vi "EC_Applied_Motion_SXSYSZ_20170419A_3chNoBK.vi"() -> ()   [LabVIEW 2015]
uses:
  <vilib>/Instr/_visa.llb/VISA Configure Serial Port (Instr).vi
  <userlib>/caLab/Private/Put_DBL-1D_PV-1D.vi
  <userlib>/caLab/Private/Put_DBL_PV.vi
  <userlib>/caLab/Private/Get_PV-1D.vi
  <vilib>/Utility/file.llb/Write To Spreadsheet File (I64).vi
  <vilib>/Utility/file.llb/Read From Spreadsheet File (I64).vi
panel:
  out "x*2^n":dbl
  out "Jog Z4-":bool
  out "Jog Z4+":bool
  in  "Jog Z-- CNTL":bool
  in  "Jog Z++ CNTL":bool
  in  "Local":bool
  out "Movex4Z REQ":bool
  in  "Reset Jog counts":bool
  in  "Jog Z- CNTL":bool
  in  "Jog Z+ CNTL":bool
  in  "Jog Y- CNTL":bool
  in  "Jog Y+ CNTL":bool
  in  "Jog X- CNTL":bool
  in  "Jog X+ CNTL":bool
  out "APX:FZ_DOWN":dbl
  out "APX:FZ_UP":dbl
  out "APX:FY_DOWN":dbl
  out "APX:FY_UP":dbl
  out "APX:FX_DOWN":dbl
  out "APX:FX_UP":dbl
  out "FZ Jog Counts In Range?":bool
  out "FY Jog Counts In Range?":bool
  out "FX Jog Counts In Range?":bool
  in  "FZ Jog counts":i8
  in  "FY Jog counts":i8
  in  "FX Jog counts":i8
  in  "Dev 5 Voltage SW":bool=TRUE
  out "Isolated from GND?":bool
  in  "Crash Override":bool
  out "Dev5 Voltage PV":dbl
  in  "APX:FZabs":dbl
  in  "Move x4Z":bool
  out "Jog Z-":bool
  out "Jog X-":bool
  out "Jog Y-":bool
  out "Z Velocity MV mm/sec":dbl format="%.3f"
  out "Z Position MV mm":dbl
  out "Y Velocity MV mm/sec":dbl format="%.3f"
  out "Y Position MV mm":dbl
  out "X Velocity MV mm/sec":dbl format="%.3f"
  out "X Position MV mm":dbl
  in  "stop":bool
  in  "Tab Control 3":enum32{"Status", "Reset"}(tab)
  out "Y in Range":bool
  out "Y in Motion":bool
  out "X  in Range":bool
  out "X  in Motion":bool
  out "Z in Range":bool
  out "Z in Motion":bool
  out "X Ready":bool
  out "Y Ready":bool
  out "Z Ready":bool
  in  "Reset Y Position mm":dbl
  out "Reset Y Motor Steps":i32
  in  "Reset X Position mm":dbl
  out "Reset X Motor Steps":i32
  in  "Reset Z Position mm":dbl
  out "Reset Z Motor Steps":i32
  in  "Reset":bool
  in  "Tab Control":enum32{"mm", "preset", "step"}(tab)
  in  "APX:FXstep":dbl=0.1 min=0.1 max=0.2
  in  "FX Velocity SP mm/sec":dbl=0.010583500000000001
  in  "APX:FYstep":dbl=0.025 min=0.025 max=0.1
  in  "FY Velocity SP mm/sec":dbl=0.010583500000000001
  in  "APX:Fzstep":dbl=0.1 min=0.05 max=0.2
  in  "FZ Velocity SP mm/sec":dbl=0.0635
  in  "Z Jog Set":bool
  in  "Y Jog Set":bool
  in  "X Jog Set":bool
  in  "X Velocity SP step/sec":i32 min=1 max=1000
  in  "Y Velocity SP step/sec":i32 min=1 max=1000
  in  "Z Velocity SP step/sec":i32 min=1 max=500
  in  "Y Step SP":i32=-20000 min=-800000 max=800000 step=500
  in  "X Step SP":i32=-20000 min=-750000 max=750000 step=500
  in  "Z Step SP":i32=-20000 min=-3000 max=102400000 step=500
  out "X Step PV":i32 max=2000
  out "Y Step PV":i32 max=2000
  out "Z Step PV":i32 max=2000
  out "R Step PV":i32 max=2000
  out "Z COM PORT":refnum<visa-resource-name>="COM5"
  out "Z Holding Current %":i32
  out "Z Run Current %":i32
  out "Z offset mm":dbl
  out "Z mm/rev":dbl
  out "Z steps/rev":u32
  out "Z  velocity PV step/sec":i32
  out "Z MINPOS":i32=-94296
  out "Z MAXPOS":i32=-34296
  out "Jog Z+":bool
  out "Z Position mm PV":dbl
  out "X Position mm PV":dbl
  out "X velocity PV step/sec":i32
  out "Jog X+":bool
  out "X Holding Current %":i32
  out "X Run Current %":i32
  out "X offset mm":dbl
  out "X mm/rev":dbl
  out "X steps/rev":u32
  out "X MAXPOS":i32=-34296
  out "X MINPOS":i32=-94296
  out "X COM PORT":refnum<visa-resource-name>="COM5"
  out "Y Holding Current %":i32
  out "Y Run Current %":i32
  out "Y Position mm PV":dbl
  out "Y offset mm":dbl
  out "Y mm/rev":dbl
  out "Y steps/rev":u32
  out "Y velocity PV step/sec":i32
  in  "Stop":bool
  out "Jog Y+":bool
  out "Y MINPOS":i32=-94296
  out "Y MAXPOS":i32=-34296
  out "Y COM PORT":refnum<visa-resource-name>="COM5"
  # "APX:FY"
  # "Sample posiitoning EPICS"
  # "x-ray"
  # "APX:FZ"
  # "APX:FX"
  # "SPEAR"
  # "APX:FinePos"
  # "Stage"
  # "Current position"
  # "Jog step/velovity"
  # "sample to SSRL"
  # "FX"
  # "FY"
  # "FZ"
  # "R,L = green"
  # "L"
  # "M"
  # "R"
  # "Preset position"
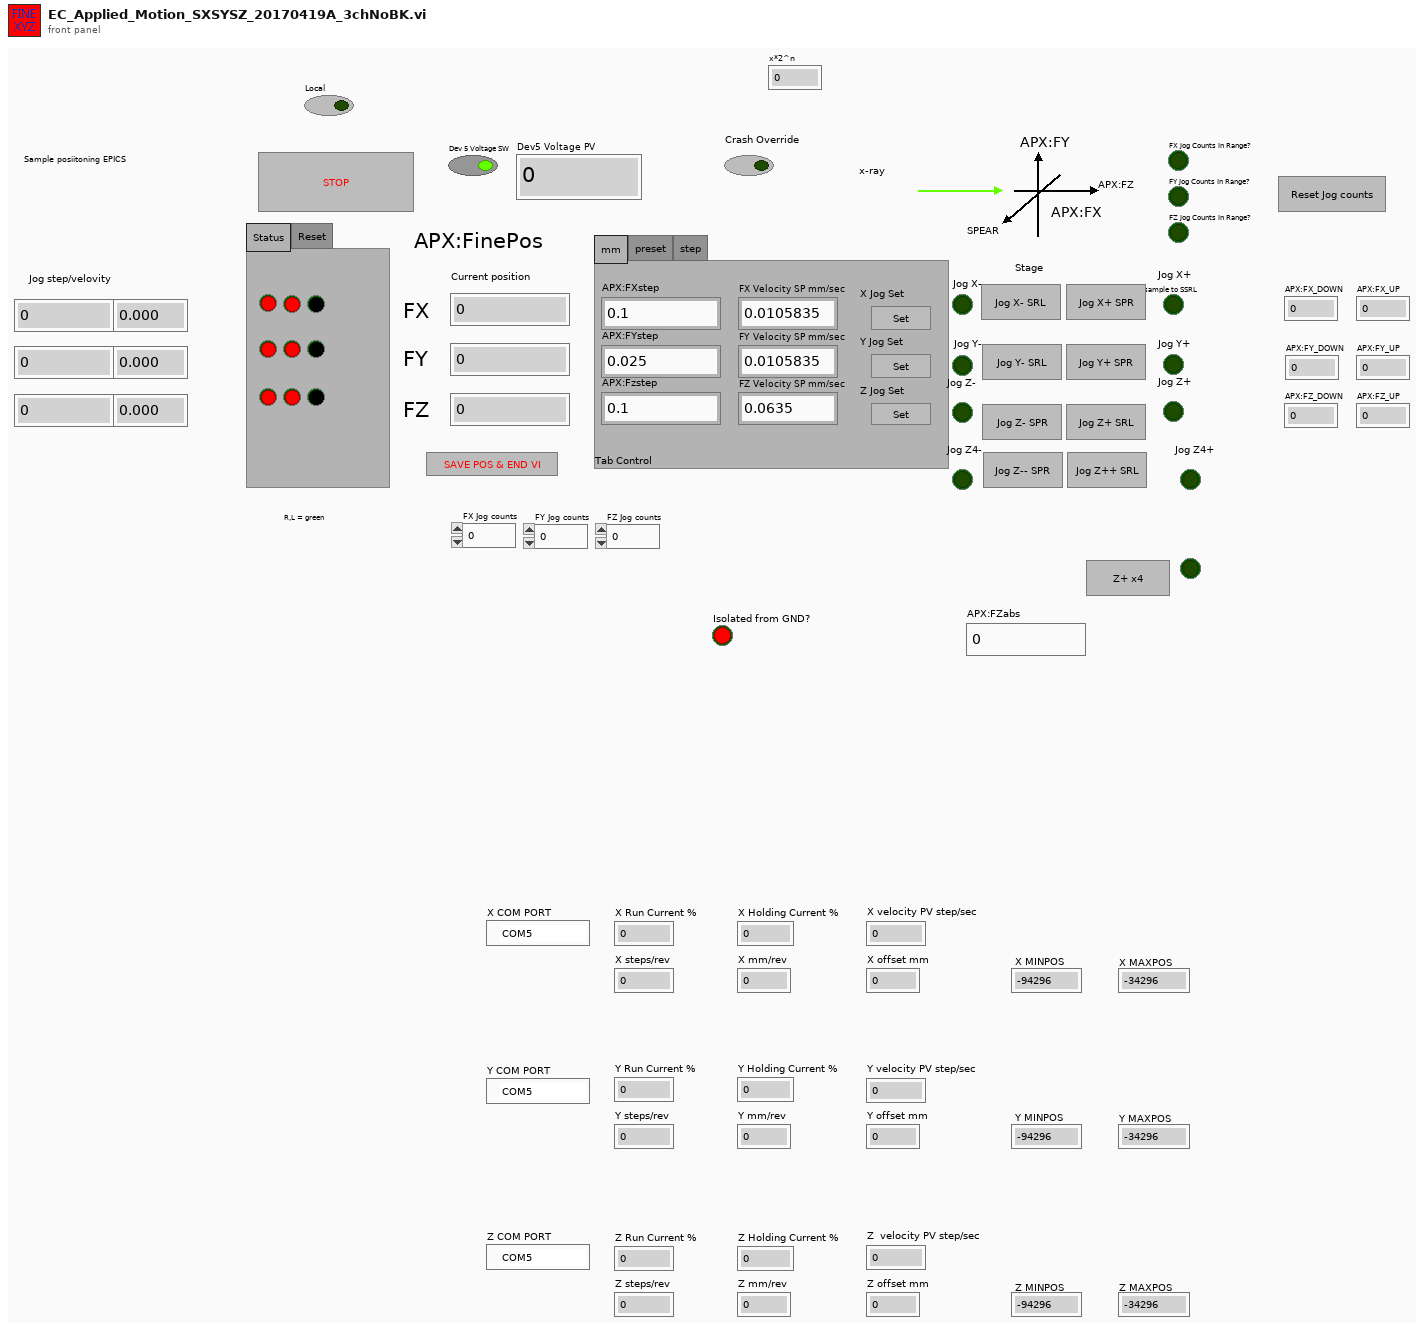
[diagram p1: front panel]
types:
  T1 = enum16{"Power-up Signature", "Accel Rate", "Accel Max", "Bit Rate", "Buffer Status", "Change Current", "Commence Jogging", "Change Jog Speed", "Continue", "Define Address", "Distance for FC,FM,FO,FY", "Decel Rate", "Distance or Position", "Define Limits", "Encoder Deadband", "Encoder Function", "Encoder Position", "Encoder Ratio", "Feed to Length with Speed Change", "Feed to Length", "Feed to Sensor with Mask Dist", "Feed to Length & Set Output", "Feed to Position", "Feed to Sensor", "Feed to Sensor w/safety", "Follow Handwheel", "Immediate Distance?", "Immediate Encoder?", "Immediate Low Output", "Immediate High Output", "Immediate Position?", "Input Status?", "Jog Accel/Decel", "Jog Disable", "Jog Enable", "Jog Speed", "Motor Disable", "Motor Enable", "Microstep Resolution", "Power up Current", "Power up Mode", "Pause", "Request Status", "Revision Level?", "Seek Home", "Stop Jogging", "Stop & Kill Buffer", "Set Output", "Set ABS Position", "Send String", "Stop", "Velocity for Speed Change", "Velocity Setting", "Wait for Input", "Wait Time"}
  T2 = enum8{"Enabled", "Disabled", "Disabled and Grayed Out"}
  T3 = cluster{"first row[0]":i64, "first row[1]":i64, "first row[2]":i64, "first row[3]":i64, "first row[4]":i64, "first row[5]":i64, "first row[6]":i64, "first row[7]":i64, "first row[8]":i64}
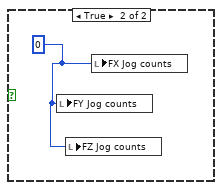
[diagram p5: hidden frame]
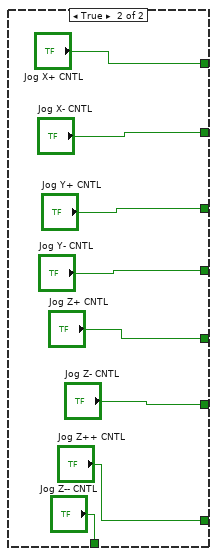
[diagram p7: hidden frame]
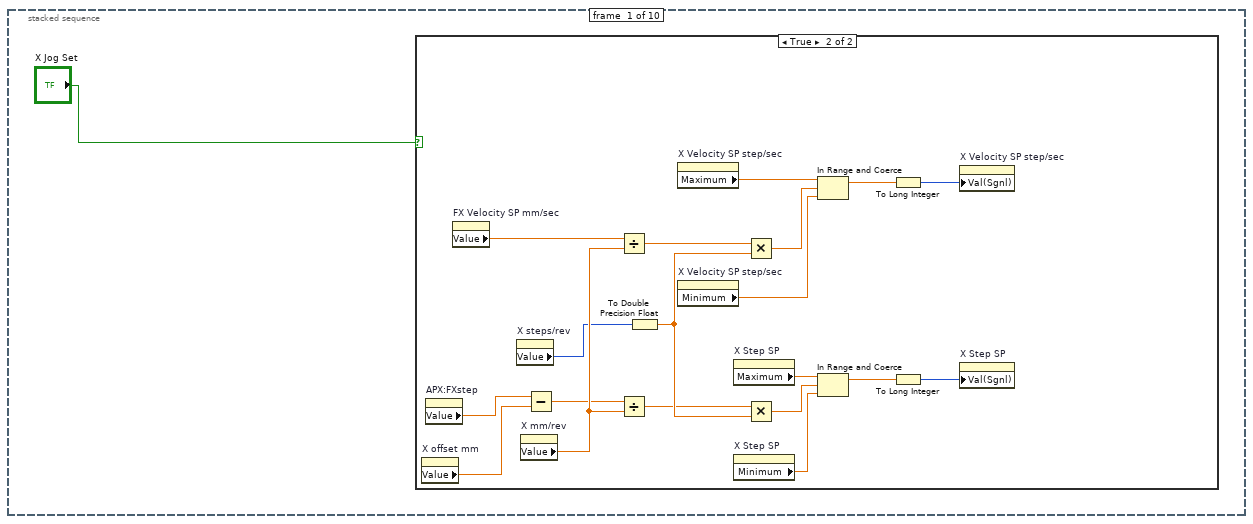
[diagram p8: hidden frame]
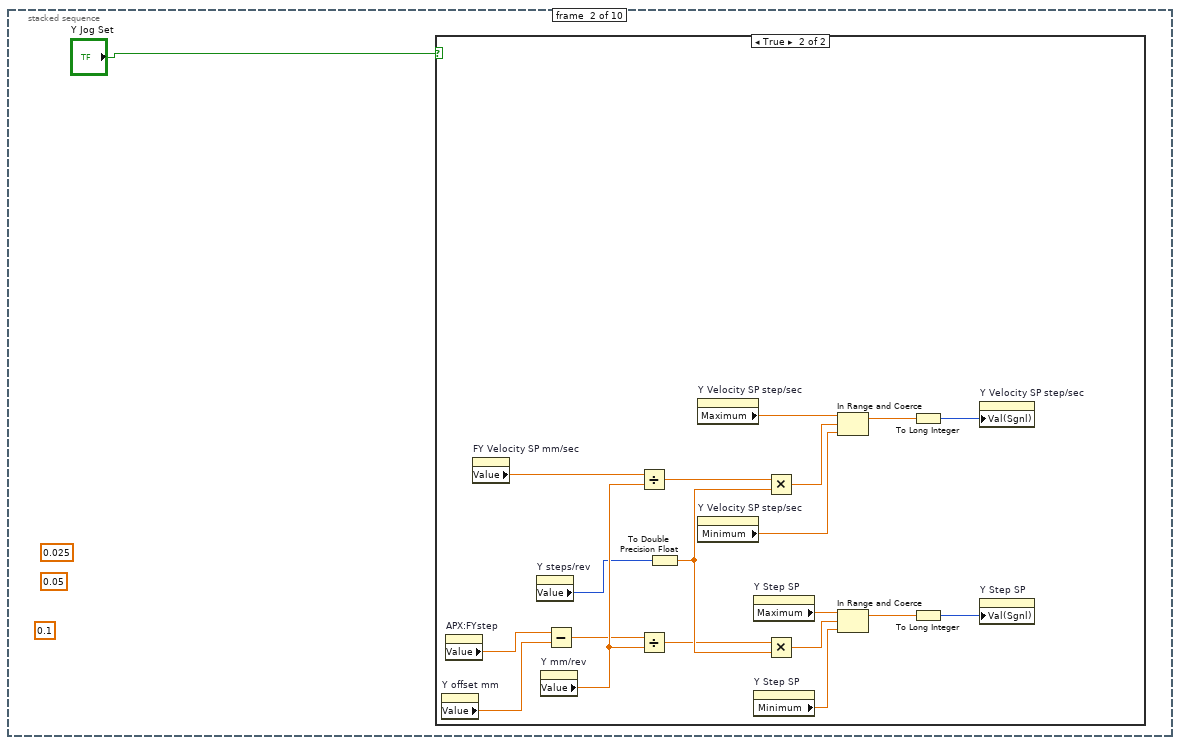
[diagram p10: hidden frame]
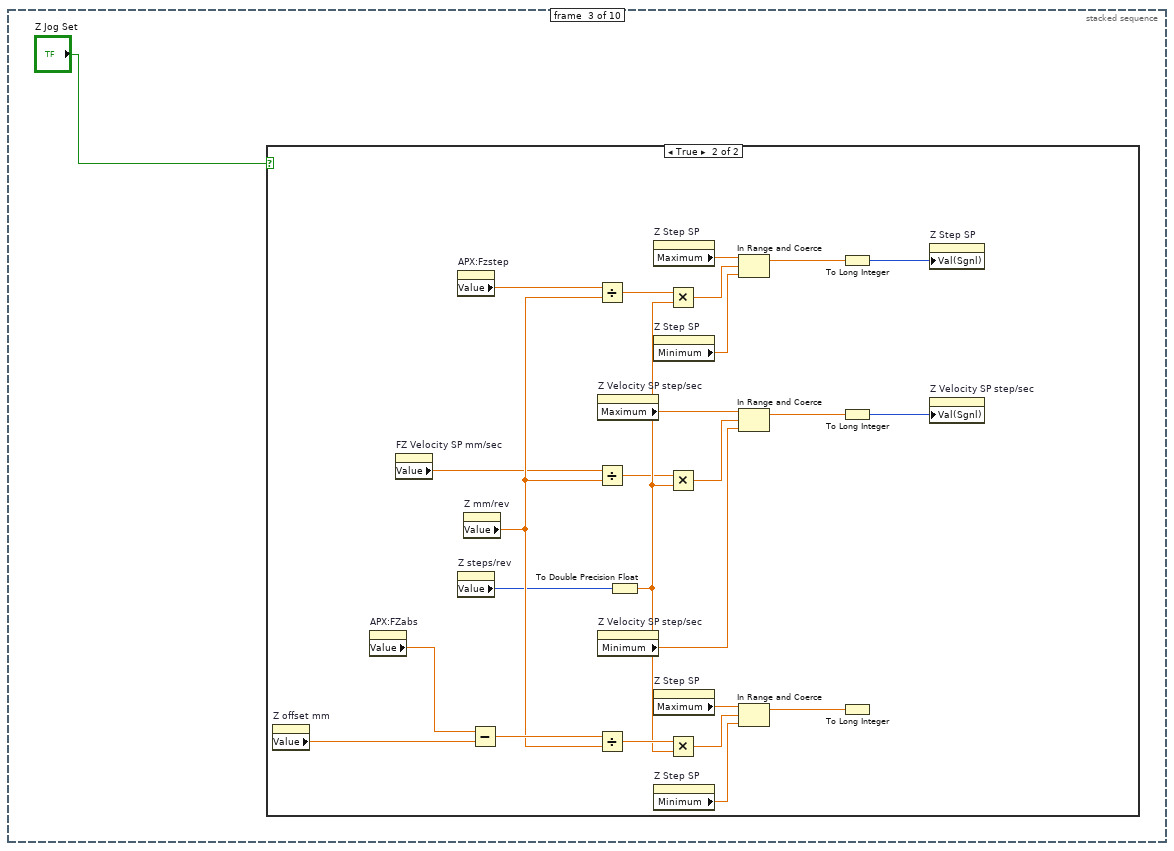
[diagram p12: hidden frame]
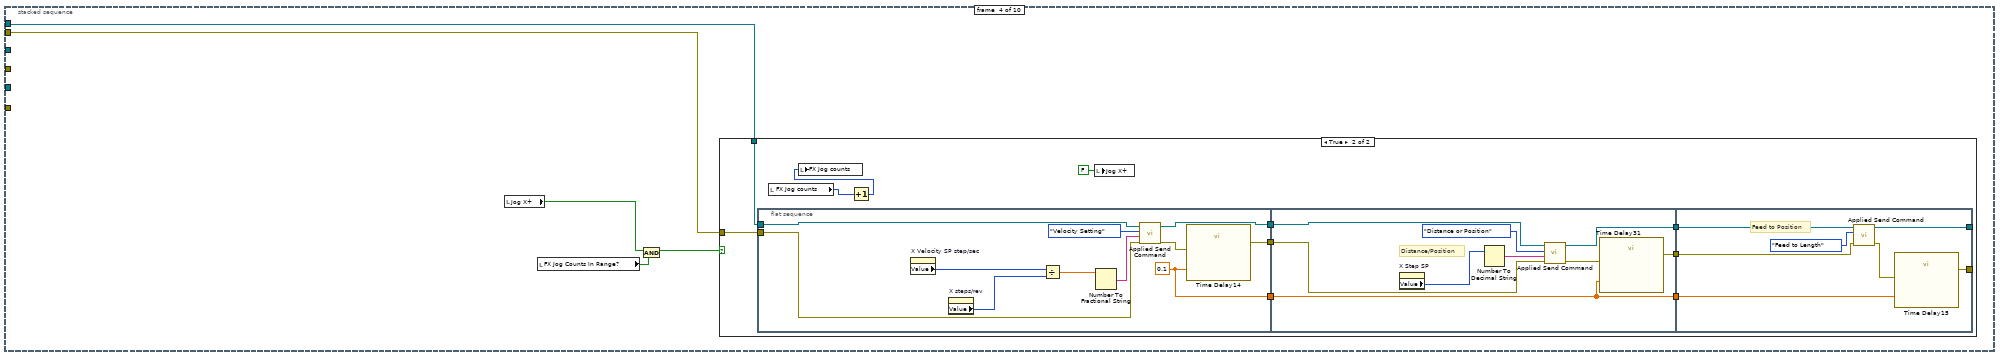
[diagram p14: hidden frame]
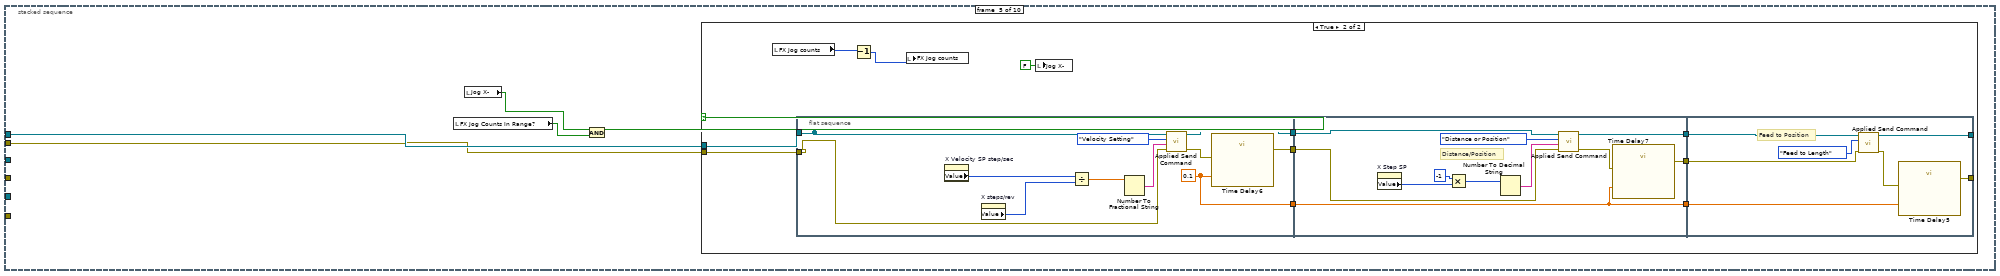
[diagram p16: hidden frame]
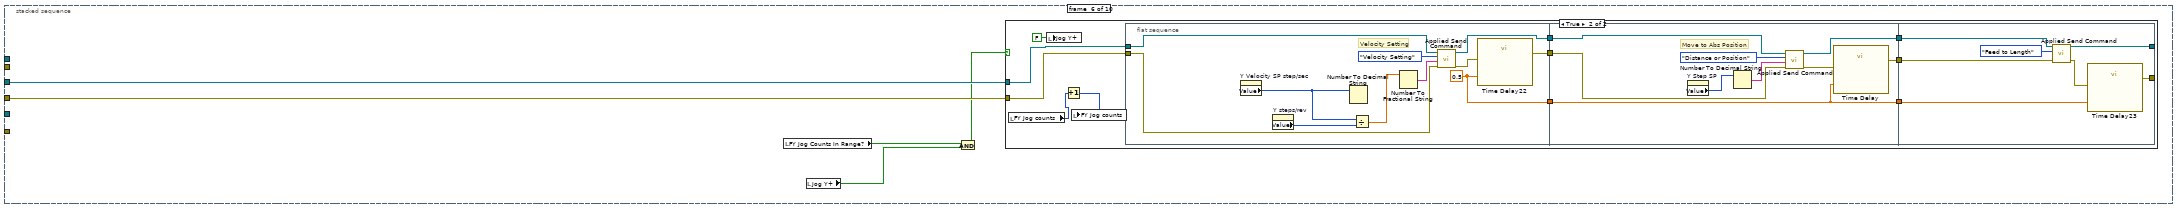
[diagram p18: hidden frame]
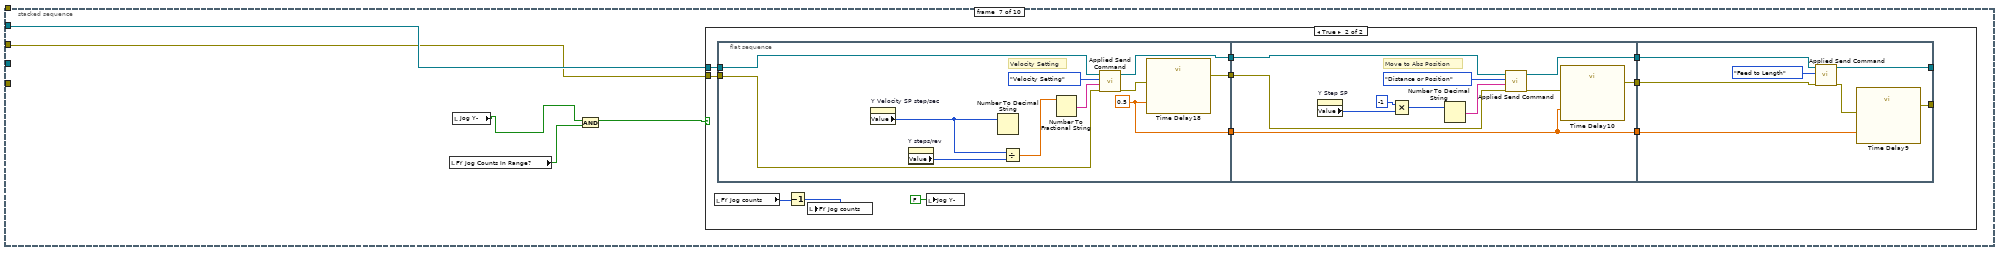
[diagram p20: hidden frame]
diagram:
  (unwired) FALSE
  n1 = flat-sequence {
    tunnel: [w58] -> w18
    tunnel: [w57] -> w17
    tunnel: w18 -> [w75]
    tunnel: w17 -> [w74]
    tunnel: [w73] -> w16
    tunnel: [w72] -> w15
    tunnel: [w78] -> w40
    tunnel: w16 -> [w86]
    tunnel: w15 -> [w85]
    tunnel: [w79] -> w14
    tunnel: w40 -> [w100]
    tunnel: [w99] -> w34
    tunnel: [w97] -> w33
    tunnel: [w102] -> w32
    tunnel: w14 -> [w101]
    tunnel: [w108] -> w38
    tunnel: [w109] -> w39
    tunnel: w34 -> [w109]
    tunnel: w33 -> [w108]
    tunnel: w32 -> [w107]
    frame #0 {
      "X Run Current %" <- 100 ("Run Current %")
      "X Holding Current %" <- 50 ("Holding Current %")
    }
    frame #1 {
      w45 = T2."Enabled" ("Disabled")
      n2 = property on="Jog X+" class="Bool"("DisabledEnum"=w45) -> ()  [unwired: 2 in, 2 out]
      n3 = property on="Jog X-" class="Bool"("DisabledEnum"=w45) -> ()  [unwired: 2 in, 2 out]
      n4 = property on="Jog Y+" class="Bool"("DisabledEnum"=w45) -> ()  [unwired: 2 in, 2 out]
      n5 = property on="Jog Z+" class="Bool"("DisabledEnum"=w45) -> ()  [unwired: 2 in, 2 out]
      n6 = property on="Jog Y-" class="Bool"("DisabledEnum"=w45) -> ()  [unwired: 2 in, 2 out]
      n7 = property on="Jog Z-" class="Bool"("DisabledEnum"=w45) -> ()  [unwired: 2 in, 2 out]
    }
    frame #2 {
      w48 = 0.21167 ("MM/rev")
      w51 = u32 20000 ("step/rev")
      w46 = 1000 ("Value (Signaling)")
      (unwired) 0.01 ("Value (Signaling)")
      n8 = property on="X Velocity SP step/sec" class="DigNum (strict)"("Minimum"=1.0 ("Data Entry Limits:Minimum")) -> ()  [unwired: 2 in, 2 out]
      n9 = property on="X Velocity SP step/sec" class="DigNum (strict)"("Val(Sgnl)"=w46) -> ()  [unwired: 2 in, 2 out]
      n10 = To Double Precision Float(number=w51) -> (double precision float=w50:dbl)
      n11 = To Double Precision Float(number=w46) -> (double precision float=w52:dbl)
      n12 = property on="X Velocity SP step/sec" class="DigNum (strict)"("Maximum"=w52) -> ()  [unwired: 2 in, 2 out]
      n13 = Divide(x=w52, y=w50) -> (x/y=w47:dbl)
      n14 = Multiply(x=w47, y=w48) -> (x*y=w49:dbl)
      n15 = property on="FX Velocity SP mm/sec" class="DigNum (strict)"("Val(Sgnl)"=w49) -> ()  [unwired: 2 in, 2 out]
      "X steps/rev" <- w51
      "X mm/rev" <- w48
    }
    frame #3 {
      w56 = -750000 ("lower limit")
      w55 = 750000 ("upper limit")
      n16 = property on="X Step SP" class="DigNum (strict)"("Maximum"=w55) -> ()  [unwired: 2 in, 2 out]
      n17 = property on="X Step SP" class="DigNum (strict)"("Minimum"=w56) -> ()  [unwired: 2 in, 2 out]
      "X offset mm" <- 0.0 ("offset")
      "X MAXPOS" <- w55
      "X MINPOS" <- w56
    }
    frame #4 {
      w65 = refnum<visa-resource-name> "COM21" ("COM PORT")
      w63 = u16 0 items=["None", "XON/XOFF", "RTS/CTS", "XON/XOFF & RTS/CTS", "DTR/DSR", "XON/XOFF & DTR/DSR"] ("flow control (0:none)")
      w62 = u16 10 items=["1.0"=10, "1.5"=15, "2.0"=20] ("stop bits (10: 1 bit)")
      # "Stop bits"
      n18 = call-poly "VISA Configure Serial Port"("VISA resource name"=w65, "timeout (10sec)"=u32 10000, "baud rate (9600)"=u32 9600, "data bits (8)"=u16 8, "parity (0:none)"=enum16{"None", "Odd", "Even", "Mark", "Space"}."None", "stop bits (10: 1 bit)"=w62, "flow control (0:none)"=w63) -> ("VISA resource name out"=w58:refnum<visa-resource-name>, "error out"=w57:errorcluster)  [unwired: 7 in]
      "X COM PORT" <- w65
    }
    frame #5 {
      n19 = property on="X Run Current" class="DigNum (strict)"() -> ("Value"=w70:i32)  [unwired: 2 in, 2 out]
      n20 = Divide(x=w70, y=100) -> (x/y=w67:dbl)
      n21 = Multiply(x=3.5 ("y"), y=w67) -> (x*y=w69:dbl)
      n22 = Number To Fractional String(number=w69) -> (F-format string=w71:string)  [unwired: 3 in]
      n23 = call "Applied Send Command.vi"("error in (no error)"=w74, "Extra"=w71, "Command"=T1."Change Current", "VISA resource name"=w75) -> ("error out"=w73:errorcluster, "VISA resource name out"=w72:refnum<visa-resource-name>)  [unwired: 3 in, 1 out]
    }
    frame #6 {
      # "VELOCITY"
      n24 = property on="X Velocity SP step/sec" class="DigNum (strict)"() -> ("Value"=w82:i32)  [unwired: 2 in, 2 out]
      n25 = property on="X steps/rev" class="DigNum (strict)"() -> ("Value"=w81:u32)  [unwired: 2 in, 2 out]
      n26 = Divide(x=w82, y=w81) -> (x/y=w80:dbl)
      n27 = Number To Fractional String(number=w80) -> (F-format string=w87:string)  [unwired: 3 in]
      n28 = call "Applied Send Command.vi"("error in (no error)"=w86, "Extra"=w87, "Command"=T1."Velocity Setting", "VISA resource name"=w85) -> ("error out"=w88:errorcluster, "VISA resource name out"=w95:refnum<visa-resource-name>)  [unwired: 3 in, 1 out]
      n29 = call "Time Delay30"("error in (no error)"=w88, "Delay Time (s)"=0.1) -> ("error out"=w93:errorcluster)  [unwired: 9 in]
      n30 = call "Applied Send Command.vi"("error in (no error)"=w93, "Extra"="", "Command"=T1."Velocity Setting", "VISA resource name"=w95) -> ("error out"=w78:errorcluster, "read buffer"=w91:string, "VISA resource name out"=w79:refnum<visa-resource-name>)  [unwired: 3 in]
      n31 = Fract/Exp String To Number(string=w91, offset=3) -> (number=w84:dbl)  [unwired: 2 in, 1 out]
      n32 = Multiply(x=w84, y=w81) -> (x*y=w83:dbl)
      n33 = property on="X velocity PV step/sec" class="DigNum (strict)"("Val(Sgnl)"=w83) -> ()  [unwired: 2 in, 2 out]
    }
    frame #7 {
      # "GET CURRENT POSITION"
      n34 = call "Applied Send Command.vi"("error in (no error)"=w100, "Extra"="", "Command"=T1."Immediate Position?", "VISA resource name"=w101) -> ("error out"=w98:errorcluster, "read buffer"=w104:string, "VISA resource name out"=w99:refnum<visa-resource-name>)  [unwired: 3 in]
      n35 = call "Time Delay13"("error in (no error)"=w98, "Delay Time (s)"=0.1) -> ("error out"=w97:errorcluster)  [unwired: 9 in]
      n36 = Hexadecimal String To Number(string=w104, offset=3) -> (number=w102:u32)  [unwired: 1 in, 1 out]
    }
    frame #8 {
      n37 = disable-structure shown="Disabled" {
        disable-tunnel: w107 -> [w110 _]
        frame Disabled {
          n38 = property on="X Step SP" class="DigNum (strict)"("Val(Sgnl)"=w110) -> ()  [unwired: 2 in, 2 out]
          n39 = property on="X Step SP" class="DigNum (strict)"() -> ("Maximum"=w113:dbl)  [unwired: 2 in, 2 out]
          n40 = property on="X Step SP" class="DigNum (strict)"() -> ("Minimum"=w112:dbl)  [unwired: 2 in, 2 out]
          n41 = In Range and Coerce(upper limit=w113, x=w110, lower limit=w112) -> (In Range?=w111:bool)  [unwired: 1 out]
          n42 = property on="X  in Range" class="Bool (strict)"("Val(Sgnl)"=w111) -> ()  [unwired: 2 in, 2 out]
        }
        frame Enabled {
        }
      }
    }
  }
  n43 = flat-sequence {
    frame #0 {
    }
    frame #1 {
      n44 = call-poly <vilib>:"Read From Spreadsheet File.vi"("file path (dialog if empty)"=path "S:/SSE/SCL2/POS.TXT") -> ("first row"=w114:i64[])  [unwired: 6 in, 4 out]
      n45 = Array To Cluster(array=w114) -> (cluster=w115:T3)
      n46 = Unbundle(w115) -> ("first row[0]"=w117:i64, "first row[1]"=w118:i64, "first row[2]"=w119:i64)  [unwired: 6 out]
      n47 = property on="Reset X Motor Steps" class="DigNum (strict)"("Val(Sgnl)"=w117) -> ()  [unwired: 2 in, 2 out]
      n48 = property on="Reset Y Motor Steps" class="DigNum (strict)"("Val(Sgnl)"=w118) -> ()  [unwired: 2 in, 2 out]
      n49 = property on="Reset Z Motor Steps" class="DigNum (strict)"("Val(Sgnl)"=w119) -> ()  [unwired: 2 in, 2 out]
    }
  }
  n50 = flat-sequence {
    tunnel: [w134] -> w5
    tunnel: [w133] -> w4
    tunnel: w5 -> [w148]
    tunnel: w4 -> [w147]
    tunnel: [w146] -> w3
    tunnel: [w145] -> w2
    tunnel: [w156] -> w31
    tunnel: [w155] -> w30
    tunnel: w3 -> [w158]
    tunnel: w2 -> [w157]
    tunnel: w31 -> [w173]
    tunnel: w30 -> [w172]
    tunnel: [w174] -> w29
    tunnel: [w175] -> w28
    tunnel: [w176] -> w1
    tunnel: [w184] -> w26
    tunnel: [w185] -> w27
    tunnel: w29 -> [w185]
    tunnel: w28 -> [w184]
    tunnel: w1 -> [w183]
    frame #0 {
      "Z Run Current %" <- 100 ("Z Run Current %")
      "Z Holding Current %" <- 50 ("Z Holding Current %")
    }
    frame #1 {
    }
    frame #2 {
      (unwired) 0.05 ("Value (Signaling)")
      w124 = 2.54 ("Z mm/rev")
      w123 = u32 20000 ("step/rev")
      w125 = 500 ("Value (Signaling)")
      n51 = property on="Z Velocity SP step/sec" class="DigNum (strict)"("Minimum"=1.0 ("Data Entry Limits:Minimum")) -> ()  [unwired: 2 in, 2 out]
      n52 = property on="Z Velocity SP step/sec" class="DigNum (strict)"("Val(Sgnl)"=w125) -> ()  [unwired: 2 in, 2 out]
      n53 = To Double Precision Float(number=w123) -> (double precision float=w128:dbl)
      n54 = To Double Precision Float(number=w125) -> (double precision float=w129:dbl)
      n55 = property on="Z Velocity SP step/sec" class="DigNum (strict)"("Maximum"=w129) -> ()  [unwired: 2 in, 2 out]
      n56 = Divide(x=w129, y=w128) -> (x/y=w126:dbl)
      n57 = Multiply(x=w126, y=w124) -> (x*y=w127:dbl)
      n58 = property on="FZ Velocity SP mm/sec" class="DigNum (strict)"("Val(Sgnl)"=w127) -> ()  [unwired: 2 in, 2 out]
      "Z mm/rev" <- w124
      "Z steps/rev" <- w123
    }
    frame #3 {
      w131 = -3000 ("lower limit")
      w130 = 102400000 ("upper limit")
      n59 = property on="Z Step SP" class="DigNum (strict)"("Minimum"=w131) -> ()  [unwired: 2 in, 2 out]
      n60 = property on="Z Step SP" class="DigNum (strict)"("Maximum"=w130) -> ()  [unwired: 2 in, 2 out]
      "Z offset mm" <- 0.0 ("Z offset mm")
      "Z MINPOS" <- w131
      "Z MAXPOS" <- w130
    }
    frame #4 {
      w141 = refnum<visa-resource-name> "COM23" ("COM PORT")
      w139 = u16 0 items=["None", "XON/XOFF", "RTS/CTS", "XON/XOFF & RTS/CTS", "DTR/DSR", "XON/XOFF & DTR/DSR"] ("flow control (0:none)")
      w138 = u16 10 items=["1.0"=10, "1.5"=15, "2.0"=20] ("stop bits (10: 1 bit)")
      # "Stop bits"
      n61 = call-poly "VISA Configure Serial Port"("VISA resource name"=w141, "timeout (10sec)"=u32 10000, "baud rate (9600)"=u32 9600, "data bits (8)"=u16 8, "parity (0:none)"=enum16{"None", "Odd", "Even", "Mark", "Space"}."None", "stop bits (10: 1 bit)"=w138, "flow control (0:none)"=w139) -> ("VISA resource name out"=w134:refnum<visa-resource-name>, "error out"=w133:errorcluster)  [unwired: 7 in]
      "Z COM PORT" <- w141
    }
    frame #5 {
      # "Run Current %"
      n62 = property on="Z Run Current %" class="DigNum (strict)"() -> ("Value"=w149:i32)  [unwired: 2 in, 2 out]
      n63 = Divide(x=w149, y=100) -> (x/y=w150:dbl)
      n64 = Multiply(x=w150, y=3.5) -> (x*y=w144:dbl)
      n65 = Number To Fractional String(number=w144) -> (F-format string=w151:string)  [unwired: 3 in]
      n66 = call "Applied Send Command.vi"("error in (no error)"=w147, "Extra"=w151, "Command"=T1."Change Current", "VISA resource name"=w148) -> ("error out"=w145:errorcluster, "VISA resource name out"=w146:refnum<visa-resource-name>)  [unwired: 3 in, 1 out]
    }
    frame #6 {
      # "VELOCITY"
      n67 = property on="Z Velocity SP step/sec" class="DigNum (strict)"() -> ("Value"=w153:i32)  [unwired: 2 in, 2 out]
      n68 = property on="Z steps/rev" class="DigNum (strict)"() -> ("Value"=w154:u32)  [unwired: 2 in, 2 out]
      n69 = Divide(x=w153, y=w154) -> (x/y=w161:dbl)
      n70 = Number To Fractional String(number=w161) -> (F-format string=w163:string)  [unwired: 3 in]
      n71 = call "Applied Send Command.vi"("error in (no error)"=w157, "Extra"=w163, "Command"=T1."Velocity Setting", "VISA resource name"=w158) -> ("error out"=w164:errorcluster, "VISA resource name out"=w171:refnum<visa-resource-name>)  [unwired: 3 in, 1 out]
      n72 = call "Time Delay2"("error in (no error)"=w164, "Delay Time (s)"=0.1) -> ("error out"=w169:errorcluster)  [unwired: 9 in]
      n73 = call "Applied Send Command.vi"("error in (no error)"=w169, "Extra"="", "Command"=T1."Velocity Setting", "VISA resource name"=w171) -> ("error out"=w155:errorcluster, "read buffer"=w167:string, "VISA resource name out"=w156:refnum<visa-resource-name>)  [unwired: 3 in]
      n74 = Fract/Exp String To Number(string=w167, offset=3) -> (number=w162:dbl)  [unwired: 2 in, 1 out]
      n75 = Multiply(x=w162, y=w154) -> (x*y=w159:dbl)
      n76 = property on="Z  velocity PV step/sec" class="DigNum (strict)"("Val(Sgnl)"=w159) -> ()  [unwired: 2 in, 2 out]
    }
    frame #7 {
      # "GET CURRENT POSITION"
      n77 = call "Applied Send Command.vi"("error in (no error)"=w172, "Extra"="", "Command"=T1."Immediate Position?", "VISA resource name"=w173) -> ("error out"=w178:errorcluster, "read buffer"=w180:string, "VISA resource name out"=w174:refnum<visa-resource-name>)  [unwired: 3 in]
      n78 = call "Time Delay8"("error in (no error)"=w178, "Delay Time (s)"=0.1) -> ("error out"=w175:errorcluster)  [unwired: 9 in]
      n79 = Hexadecimal String To Number(string=w180, offset=3) -> (number=w176:u32)  [unwired: 1 in, 1 out]
    }
    frame #8 {
      n80 = disable-structure shown="Disabled" {
        disable-tunnel: w183 -> [w188 _]
        frame Disabled {
          n81 = property on="Z Step SP" class="DigNum (strict)"("Val(Sgnl)"=w188) -> ()  [unwired: 2 in, 2 out]
          n82 = property on="Z Step SP" class="DigNum (strict)"() -> ("Maximum"=w187:dbl)  [unwired: 2 in, 2 out]
          n83 = property on="Z Step SP" class="DigNum (strict)"() -> ("Minimum"=w186:dbl)  [unwired: 2 in, 2 out]
          n84 = In Range and Coerce(upper limit=w187, x=w188, lower limit=w186) -> (In Range?=w189:bool)  [unwired: 1 out]
          n85 = property on="Z in Range" class="Bool (strict)"("Val(Sgnl)"=w189) -> ()  [unwired: 2 in, 2 out]
        }
        frame Enabled {
        }
      }
    }
  }
  n86 = flat-sequence {
    tunnel: [w204] -> w13
    tunnel: [w203] -> w12
    tunnel: w13 -> [w218]
    tunnel: w12 -> [w217]
    tunnel: [w216] -> w11
    tunnel: [w215] -> w10
    tunnel: w11 -> [w226]
    tunnel: w10 -> [w225]
    tunnel: [w224] -> w9
    tunnel: [w223] -> w8
    tunnel: [w243] -> w35
    tunnel: w9 -> [w246]
    tunnel: w8 -> [w245]
    tunnel: [w244] -> w7
    tunnel: [w242] -> w6
    tunnel: [w253] -> w41
    tunnel: [w255] -> w42
    tunnel: w35 -> [w253]
    tunnel: w7 -> [w255]
    tunnel: w6 -> [w254]
    frame #0 {
      "Y Run Current %" <- 100 ("Run Current %")
      "Y Holding Current %" <- 50 ("Holding Current %")
    }
    frame #1 {
    }
    frame #2 {
      w194 = 0.21167 ("MM/rev")
      w197 = u32 20000 ("step/rev")
      w192 = 1000 ("Value (Signaling)")
      (unwired) 0.01 ("Value (Signaling)")
      n87 = property on="Y Velocity SP step/sec" class="DigNum (strict)"("Minimum"=1.0 ("Data Entry Limits:Minimum")) -> ()  [unwired: 2 in, 2 out]
      n88 = property on="Y Velocity SP step/sec" class="DigNum (strict)"("Val(Sgnl)"=w192) -> ()  [unwired: 2 in, 2 out]
      n89 = To Double Precision Float(number=w197) -> (double precision float=w196:dbl)
      n90 = To Double Precision Float(number=w192) -> (double precision float=w198:dbl)
      n91 = property on="Y Velocity SP step/sec" class="DigNum (strict)"("Maximum"=w198) -> ()  [unwired: 2 in, 2 out]
      n92 = Divide(x=w198, y=w196) -> (x/y=w193:dbl)
      n93 = Multiply(x=w193, y=w194) -> (x*y=w195:dbl)
      n94 = property on="FY Velocity SP mm/sec" class="DigNum (strict)"("Val(Sgnl)"=w195) -> ()  [unwired: 2 in, 2 out]
      "Y steps/rev" <- w197
      "Y mm/rev" <- w194
    }
    frame #3 {
      w201 = -800000 ("lower limit")
      w202 = 800000 ("upper limit")
      n95 = property on="Y Step SP" class="DigNum (strict)"("Maximum"=w202) -> ()  [unwired: 2 in, 2 out]
      n96 = property on="Y Step SP" class="DigNum (strict)"("Minimum"=w201) -> ()  [unwired: 2 in, 2 out]
      "Y MAXPOS" <- w202
      "Y MINPOS" <- w201
      "Y offset mm" <- 0.0 ("offset")
    }
    frame #4 {
      w211 = refnum<visa-resource-name> "COM22" ("COM PORT")
      w209 = u16 0 items=["None", "XON/XOFF", "RTS/CTS", "XON/XOFF & RTS/CTS", "DTR/DSR", "XON/XOFF & DTR/DSR"] ("flow control (0:none)")
      w208 = u16 10 items=["1.0"=10, "1.5"=15, "2.0"=20] ("stop bits (10: 1 bit)")
      # "Stop bits"
      n97 = call-poly "VISA Configure Serial Port"("VISA resource name"=w211, "timeout (10sec)"=u32 10000, "baud rate (9600)"=u32 9600, "data bits (8)"=u16 8, "parity (0:none)"=enum16{"None", "Odd", "Even", "Mark", "Space"}."None", "stop bits (10: 1 bit)"=w208, "flow control (0:none)"=w209) -> ("VISA resource name out"=w204:refnum<visa-resource-name>, "error out"=w203:errorcluster)  [unwired: 7 in]
      "Y COM PORT" <- w211
    }
    frame #5 {
      n98 = property on="Y Run Current %" class="DigNum (strict)"() -> ("Value"=w219:i32)  [unwired: 2 in, 2 out]
      n99 = Divide(x=w219, y=100) -> (x/y=w220:dbl)
      n100 = Multiply(x=w220, y=3.5) -> (x*y=w214:dbl)
      n101 = Number To Fractional String(number=w214) -> (F-format string=w221:string)  [unwired: 3 in]
      n102 = call "Applied Send Command.vi"("error in (no error)"=w217, "Extra"=w221, "Command"=T1."Change Current", "VISA resource name"=w218) -> ("error out"=w215:errorcluster, "VISA resource name out"=w216:refnum<visa-resource-name>)  [unwired: 3 in, 1 out]
    }
    frame #6 {
      # "VELOCITY"
      n103 = property on="Y Velocity SP step/sec" class="DigNum (strict)"() -> ("Value"=w227:i32)  [unwired: 2 in, 2 out]
      n104 = property on="Y steps/rev" class="DigNum (strict)"() -> ("Value"=w230:u32)  [unwired: 2 in, 2 out]
      n105 = Divide(x=w227, y=w230) -> (x/y=w229:dbl)
      n106 = Number To Fractional String(number=w229) -> (F-format string=w233:string)  [unwired: 3 in]
      n107 = call "Applied Send Command.vi"("error in (no error)"=w225, "Extra"=w233, "Command"=T1."Velocity Setting", "VISA resource name"=w226) -> ("error out"=w234:errorcluster, "VISA resource name out"=w241:refnum<visa-resource-name>)  [unwired: 3 in, 1 out]
      n108 = call "Time Delay36"("error in (no error)"=w234, "Delay Time (s)"=0.1) -> ("error out"=w239:errorcluster)  [unwired: 9 in]
      n109 = call "Applied Send Command.vi"("error in (no error)"=w239, "Extra"="", "Command"=T1."Velocity Setting", "VISA resource name"=w241) -> ("error out"=w223:errorcluster, "read buffer"=w237:string, "VISA resource name out"=w224:refnum<visa-resource-name>)  [unwired: 3 in]
      n110 = Fract/Exp String To Number(string=w237, offset=3) -> (number=w232:dbl)  [unwired: 2 in, 1 out]
      n111 = Multiply(x=w232, y=w230) -> (x*y=w231:dbl)
      n112 = property on="Y velocity PV step/sec" class="DigNum (strict)"("Val(Sgnl)"=w231) -> ()  [unwired: 2 in, 2 out]
    }
    frame #7 {
      # "GET CURRENT POSITION"
      n113 = call "Applied Send Command.vi"("error in (no error)"=w245, "Extra"="", "Command"=T1."Immediate Position?", "VISA resource name"=w246) -> ("error out"=w248:errorcluster, "read buffer"=w250:string, "VISA resource name out"=w244:refnum<visa-resource-name>)  [unwired: 3 in]
      n114 = call "Time Delay37"("error in (no error)"=w248, "Delay Time (s)"=0.1) -> ("error out"=w243:errorcluster)  [unwired: 9 in]
      n115 = Hexadecimal String To Number(string=w250, offset=3) -> (number=w242:u32)  [unwired: 1 in, 1 out]
    }
    frame #8 {
      n116 = disable-structure shown="Disabled" {
        disable-tunnel: w254 -> [w258 _]
        frame Disabled {
          n117 = property on="Y Step SP" class="DigNum (strict)"("Val(Sgnl)"=w258) -> ()  [unwired: 2 in, 2 out]
          n118 = property on="Y Step SP" class="DigNum (strict)"() -> ("Maximum"=w257:dbl)  [unwired: 2 in, 2 out]
          n119 = property on="Y Step SP" class="DigNum (strict)"() -> ("Minimum"=w256:dbl)  [unwired: 2 in, 2 out]
          n120 = In Range and Coerce(upper limit=w257, x=w258, lower limit=w256) -> (In Range?=w259:bool)  [unwired: 1 out]
          n121 = property on="Y in Range" class="Bool (strict)"("Val(Sgnl)"=w259) -> ()  [unwired: 2 in, 2 out]
        }
        frame Enabled {
        }
      }
    }
  }
  n122 = while {
    tunnel: w42 -> [w276]
    tunnel: w41 -> [w275]
    tunnel: [w296] -> w22
    tunnel: [w295] -> w23
    tunnel: w39 -> [w278]
    tunnel: w38 -> [w277]
    tunnel: [w293] -> w37
    tunnel: [w292] -> w36
    tunnel: w27 -> [w274]
    tunnel: w26 -> [w273]
    tunnel: [w291] -> w25
    tunnel: [w290] -> w24
    tunnel: [w289] -> _
    tunnel: [w288] -> _
    stop <- "stop" stop-if-true
    n123 = flat-sequence {
      frame #0 {
      }
      frame #1 {
      }
    }
    n124 = flat-sequence {
      frame #0 {
      }
      frame #1 {
      }
    }
    n125 = local read "X Position mm PV"() -> (w285:dbl)
    n126 = local read "Y Position mm PV"() -> (w284:dbl)
    n127 = local read "Z Position mm PV"() -> (w286:dbl)
    n128 = local read "FZ Jog counts"() -> (w262:i8)
    n129 = local read "FY Jog counts"() -> (w266:i8)
    n130 = local read "FX Jog counts"() -> (w270:i8)
    n131 = Build Array("APX:PiezeX", "APX:PiezeY", "APX:PiezeZ") -> (w280:string[])
    n132 = Build Array(w285, w284, w286) -> (w279:dbl[])
    n133 = call-poly <userlib>:"CaLabPut.vi"("Values"=w279, "PV Names"=w280) -> ()  [unwired: 6 in, 4 out]
    n134 = In Range and Coerce(upper limit=10.0, x=w270, lower limit=-10.0) -> (In Range?=→"FX Jog Counts In Range?":bool)  [unwired: 1 out]
    n135 = In Range and Coerce(upper limit=4.0, x=w266, lower limit=-4.0) -> (In Range?=→"FY Jog Counts In Range?":bool)  [unwired: 1 out]
    n136 = In Range and Coerce(upper limit=20.0, x=w262, lower limit=-2.0) -> (In Range?=→"FZ Jog Counts In Range?":bool)  [unwired: 1 out]
    n137 = stacked-sequence {
      tunnel: w278 -> [_ _ _ w456 w499 _ _ _ _ _]
      tunnel: w277 -> [_ _ _ w455 w498 _ _ _ _ _]
      tunnel: w276 -> [_ _ _ _ _ w544 w587 _ _ _]
      tunnel: w275 -> [_ _ _ _ _ w543 w586 _ _ _]
      tunnel: w274 -> [_ _ _ _ _ _ _ w632 w675 w719]
      tunnel: w273 -> [_ _ _ _ _ _ _ w631 w674 w720]
      frame #0 {
        n138 = case shown="True" "X Jog Set" {
          frame False {
          }
          frame True {
            n139 = property on="X offset mm" class="DigNum (strict)"() -> ("Value"=w391:dbl)  [unwired: 2 in, 2 out]
            n140 = property on="APX:FXstep" class="DigNum (strict)"() -> ("Value"=w392:dbl)  [unwired: 2 in, 2 out]
            n141 = property on="FX Velocity SP mm/sec" class="DigNum (strict)"() -> ("Value"=w398:dbl)  [unwired: 2 in, 2 out]
            n142 = property on="X steps/rev" class="DigNum (strict)"() -> ("Value"=w389:u32)  [unwired: 2 in, 2 out]
            n143 = property on="X mm/rev" class="DigNum (strict)"() -> ("Value"=w405:dbl)  [unwired: 2 in, 2 out]
            n144 = Subtract(x=w392, y=w391) -> (x-y=w388:dbl)
            n145 = Divide(x=w398, y=w405) -> (x/y=w397:dbl)
            n146 = Divide(x=w388, y=w405) -> (x/y=w387:dbl)
            n147 = To Double Precision Float(number=w389) -> (double precision float=w404:dbl)
            n148 = property on="X Velocity SP step/sec" class="DigNum (strict)"() -> ("Maximum"=w402:dbl)  [unwired: 2 in, 2 out]
            n149 = property on="X Velocity SP step/sec" class="DigNum (strict)"() -> ("Minimum"=w403:dbl)  [unwired: 2 in, 2 out]
            n150 = property on="X Step SP" class="DigNum (strict)"() -> ("Maximum"=w395:dbl)  [unwired: 2 in, 2 out]
            n151 = property on="X Step SP" class="DigNum (strict)"() -> ("Minimum"=w396:dbl)  [unwired: 2 in, 2 out]
            n152 = Multiply(x=w397, y=w404) -> (x*y=w400:dbl)
            n153 = Multiply(x=w387, y=w404) -> (x*y=w393:dbl)
            n154 = In Range and Coerce(upper limit=w402, x=w400, lower limit=w403) -> (coerced(x)=w401:dbl)  [unwired: 1 out]
            n155 = In Range and Coerce(upper limit=w395, x=w393, lower limit=w396) -> (coerced(x)=w394:dbl)  [unwired: 1 out]
            n156 = To Long Integer(number=w401) -> (32bit integer=w399:i32)
            n157 = To Long Integer(number=w394) -> (32bit integer=w390:i32)
            n158 = property on="X Velocity SP step/sec" class="DigNum (strict)"("Val(Sgnl)"=w399) -> ()  [unwired: 2 in, 2 out]
            n159 = property on="X Step SP" class="DigNum (strict)"("Val(Sgnl)"=w390) -> ()  [unwired: 2 in, 2 out]
          }
        }
      }
      frame #1 {
        (unwired) 0.1
        (unwired) 0.05
        (unwired) 0.025
        n160 = case shown="True" "Y Jog Set" {
          frame False {
          }
          frame True {
            n161 = property on="Y offset mm" class="DigNum (strict)"() -> ("Value"=w411:dbl)  [unwired: 2 in, 2 out]
            n162 = property on="APX:FYstep" class="DigNum (strict)"() -> ("Value"=w412:dbl)  [unwired: 2 in, 2 out]
            n163 = property on="FY Velocity SP mm/sec" class="DigNum (strict)"() -> ("Value"=w418:dbl)  [unwired: 2 in, 2 out]
            n164 = property on="Y steps/rev" class="DigNum (strict)"() -> ("Value"=w409:u32)  [unwired: 2 in, 2 out]
            n165 = property on="Y mm/rev" class="DigNum (strict)"() -> ("Value"=w425:dbl)  [unwired: 2 in, 2 out]
            n166 = Subtract(x=w412, y=w411) -> (x-y=w408:dbl)
            n167 = Divide(x=w418, y=w425) -> (x/y=w417:dbl)
            n168 = Divide(x=w408, y=w425) -> (x/y=w407:dbl)
            n169 = To Double Precision Float(number=w409) -> (double precision float=w424:dbl)
            n170 = property on="Y Velocity SP step/sec" class="DigNum (strict)"() -> ("Maximum"=w422:dbl)  [unwired: 2 in, 2 out]
            n171 = property on="Y Velocity SP step/sec" class="DigNum (strict)"() -> ("Minimum"=w423:dbl)  [unwired: 2 in, 2 out]
            n172 = property on="Y Step SP" class="DigNum (strict)"() -> ("Maximum"=w415:dbl)  [unwired: 2 in, 2 out]
            n173 = property on="Y Step SP" class="DigNum (strict)"() -> ("Minimum"=w416:dbl)  [unwired: 2 in, 2 out]
            n174 = Multiply(x=w417, y=w424) -> (x*y=w420:dbl)
            n175 = Multiply(x=w407, y=w424) -> (x*y=w413:dbl)
            n176 = In Range and Coerce(upper limit=w422, x=w420, lower limit=w423) -> (coerced(x)=w421:dbl)  [unwired: 1 out]
            n177 = In Range and Coerce(upper limit=w415, x=w413, lower limit=w416) -> (coerced(x)=w414:dbl)  [unwired: 1 out]
            n178 = To Long Integer(number=w421) -> (32bit integer=w419:i32)
            n179 = To Long Integer(number=w414) -> (32bit integer=w410:i32)
            n180 = property on="Y Velocity SP step/sec" class="DigNum (strict)"("Val(Sgnl)"=w419) -> ()  [unwired: 2 in, 2 out]
            n181 = property on="Y Step SP" class="DigNum (strict)"("Val(Sgnl)"=w410) -> ()  [unwired: 2 in, 2 out]
          }
        }
      }
      frame #2 {
        n182 = case shown="True" "Z Jog Set" {
          frame False {
          }
          frame True {
            n183 = property on="Z offset mm" class="DigNum (strict)"() -> ("Value"=w449:dbl)  [unwired: 2 in, 2 out]
            n184 = property on="APX:FZabs" class="DigNum (strict)"() -> ("Value"=w451:dbl)  [unwired: 2 in, 2 out]
            n185 = property on="FZ Velocity SP mm/sec" class="DigNum (strict)"() -> ("Value"=w436:dbl)  [unwired: 2 in, 2 out]
            n186 = property on="APX:Fzstep" class="DigNum (strict)"() -> ("Value"=w430:dbl)  [unwired: 2 in, 2 out]
            n187 = property on="Z steps/rev" class="DigNum (strict)"() -> ("Value"=w428:u32)  [unwired: 2 in, 2 out]
            n188 = property on="Z mm/rev" class="DigNum (strict)"() -> ("Value"=w448:dbl)  [unwired: 2 in, 2 out]
            n189 = Subtract(x=w451, y=w449) -> (x-y=w450:dbl)
            n190 = Divide(x=w430, y=w448) -> (x/y=w427:dbl)
            n191 = Divide(x=w436, y=w448) -> (x/y=w435:dbl)
            n192 = Divide(x=w450, y=w448) -> (x/y=w447:dbl)
            n193 = property on="Z Velocity SP step/sec" class="DigNum (strict)"() -> ("Maximum"=w440:dbl)  [unwired: 2 in, 2 out]
            n194 = property on="Z Velocity SP step/sec" class="DigNum (strict)"() -> ("Minimum"=w441:dbl)  [unwired: 2 in, 2 out]
            n195 = To Double Precision Float(number=w428) -> (double precision float=w446:dbl)
            n196 = property on="Z Step SP" class="DigNum (strict)"() -> ("Maximum"=w433:dbl)  [unwired: 2 in, 2 out]
            n197 = property on="Z Step SP" class="DigNum (strict)"() -> ("Minimum"=w434:dbl)  [unwired: 2 in, 2 out]
            n198 = property on="Z Step SP" class="DigNum (strict)"() -> ("Maximum"=w443:dbl)  [unwired: 2 in, 2 out]
            n199 = property on="Z Step SP" class="DigNum (strict)"() -> ("Minimum"=w444:dbl)  [unwired: 2 in, 2 out]
            n200 = Multiply(x=w427, y=w446) -> (x*y=w431:dbl)
            n201 = Multiply(x=w435, y=w446) -> (x*y=w438:dbl)
            n202 = Multiply(x=w447, y=w446) -> (x*y=w445:dbl)
            n203 = In Range and Coerce(upper limit=w433, x=w431, lower limit=w434) -> (coerced(x)=w432:dbl)  [unwired: 1 out]
            n204 = In Range and Coerce(upper limit=w440, x=w438, lower limit=w441) -> (coerced(x)=w439:dbl)  [unwired: 1 out]
            n205 = In Range and Coerce(upper limit=w443, x=w445, lower limit=w444) -> (coerced(x)=w442:dbl)  [unwired: 1 out]
            n206 = To Long Integer(number=w432) -> (32bit integer=w429:i32)
            n207 = To Long Integer(number=w439) -> (32bit integer=w437:i32)
            n208 = To Long Integer(number=w442) -> ()  [unwired: 1 out]
            n209 = property on="Z Step SP" class="DigNum (strict)"("Val(Sgnl)"=w429) -> ()  [unwired: 2 in, 2 out]
            n210 = property on="Z Velocity SP step/sec" class="DigNum (strict)"("Val(Sgnl)"=w437) -> ()  [unwired: 2 in, 2 out]
          }
        }
      }
      frame #3 {
        n211 = local read "Jog X+"() -> (w452:bool)
        n212 = local read "FX Jog Counts In Range?"() -> (w453:bool)
        n213 = And(x=w452, y=w453) -> (x .and. y?=w454:bool)
        n214 = case shown="True" w454 {
          tunnel: w456 -> [_ w461]
          tunnel: w455 -> [_ w460]
          frame False {
          }
          frame True {
            n215 = flat-sequence {
              tunnel: [w472] -> w467
              tunnel: [w469] -> w466
              tunnel: [w468] -> w465
              tunnel: w461 -> [w474]
              tunnel: w460 -> [w473]
              tunnel: w467 -> [w481]
              tunnel: [w480] -> w464
              tunnel: w466 -> [w482]
              tunnel: [w483] -> w463
              tunnel: w465 -> [w479]
              tunnel: [w479] -> w462
              tunnel: w464 -> [w494]
              tunnel: w463 -> [w493]
              tunnel: [w492] -> _
              tunnel: [w491] -> _
              tunnel: w462 -> [w490]
              frame #0 {
                w468 = 0.1 ("Delay Time (s)")
                n216 = property on="X Velocity SP step/sec" class="DigNum (strict)"() -> ("Value"=w471:i32)  [unwired: 2 in, 2 out]
                n217 = property on="X steps/rev" class="DigNum (strict)"() -> ("Value"=w475:u32)  [unwired: 2 in, 2 out]
                n218 = Divide(x=w471, y=w475) -> (x/y=w476:dbl)
                n219 = Number To Fractional String(number=w476) -> (F-format string=w477:string)  [unwired: 3 in]
                n220 = call "Applied Send Command.vi"("error in (no error)"=w473, "Extra"=w477, "Command"=T1."Velocity Setting", "VISA resource name"=w474) -> ("error out"=w470:errorcluster, "VISA resource name out"=w472:refnum<visa-resource-name>)  [unwired: 3 in, 1 out]
                n221 = call "Time Delay14"("error in (no error)"=w470, "Delay Time (s)"=w468) -> ("error out"=w469:errorcluster)  [unwired: 9 in]
              }
              frame #1 {
                # "Distance/Position"
                n222 = property on="X Step SP" class="DigNum (strict)"() -> ("Value"=w484:i32)  [unwired: 2 in, 2 out]
                n223 = Number To Decimal String(number=w484) -> (decimal integer string=w486:string)  [unwired: 1 in]
                n224 = call "Applied Send Command.vi"("error in (no error)"=w482, "Extra"=w486, "Command"=T1."Distance or Position", "VISA resource name"=w481) -> ("error out"=w485:errorcluster, "VISA resource name out"=w480:refnum<visa-resource-name>)  [unwired: 3 in, 1 out]
                n225 = call "Time Delay31"("error in (no error)"=w485, "Delay Time (s)"=w479) -> ("error out"=w483:errorcluster)  [unwired: 9 in]
              }
              frame #2 {
                # "Feed to Position"
                n226 = call "Applied Send Command.vi"("error in (no error)"=w493, "Command"=T1."Feed to Length", "VISA resource name"=w494) -> ("error out"=w488:errorcluster, "VISA resource name out"=w492:refnum<visa-resource-name>)  [unwired: 4 in, 1 out]
                n227 = call "Time Delay15"("error in (no error)"=w488, "Delay Time (s)"=w490) -> ("error out"=w491:errorcluster)  [unwired: 9 in]
              }
            }
            n228 = local read "FX Jog counts"() -> (w459:i8)
            n229 = Increment(x=w459) -> (x+1=w458:i8)
            n230 = local write "FX Jog counts"(w458) -> ()
            n231 = local write "Jog X+"(FALSE ("Jog X+")) -> ()
          }
        }
      }
      frame #4 {
        n232 = local read "FX Jog Counts In Range?"() -> (w496:bool)
        n233 = local read "Jog X-"() -> (w495:bool)
        n234 = And(x=w495, y=w496) -> (x .and. y?=w497:bool)
        n235 = case shown="True" w497 {
          tunnel: w499 -> [_ w504]
          tunnel: w498 -> [_ w503]
          frame False {
          }
          frame True {
            n236 = local read "FX Jog counts"() -> (w502:i8)
            n237 = flat-sequence {
              tunnel: [w517] -> w510
              tunnel: [w514] -> w509
              tunnel: [w513] -> w508
              tunnel: [w512] -> _
              tunnel: w504 -> [w512]
              tunnel: w503 -> [w511]
              tunnel: w510 -> [w526]
              tunnel: [w525] -> w507
              tunnel: w509 -> [w527]
              tunnel: [w528] -> w506
              tunnel: w508 -> [w524]
              tunnel: [w524] -> w505
              tunnel: w507 -> [w539]
              tunnel: w506 -> [w538]
              tunnel: [w537] -> _
              tunnel: [w536] -> _
              tunnel: w505 -> [w535]
              frame #0 {
                w513 = 0.1 ("Delay Time (s)")
                n238 = property on="X Velocity SP step/sec" class="DigNum (strict)"() -> ("Value"=w516:i32)  [unwired: 2 in, 2 out]
                n239 = property on="X steps/rev" class="DigNum (strict)"() -> ("Value"=w518:u32)  [unwired: 2 in, 2 out]
                n240 = Divide(x=w516, y=w518) -> (x/y=w519:dbl)
                n241 = Number To Fractional String(number=w519) -> (F-format string=w520:string)  [unwired: 3 in]
                n242 = call "Applied Send Command.vi"("error in (no error)"=w511, "Extra"=w520, "Command"=T1."Velocity Setting", "VISA resource name"=w512) -> ("error out"=w515:errorcluster, "VISA resource name out"=w517:refnum<visa-resource-name>)  [unwired: 3 in, 1 out]
                n243 = call "Time Delay6"("error in (no error)"=w515, "Delay Time (s)"=w513) -> ("error out"=w514:errorcluster)  [unwired: 9 in]
              }
              frame #1 {
                # "Distance/Position"
                n244 = property on="X Step SP" class="DigNum (strict)"() -> ("Value"=w529:i32)  [unwired: 2 in, 2 out]
                n245 = Multiply(x=-1, y=w529) -> (x*y=w523:i32)
                n246 = Number To Decimal String(number=w523) -> (decimal integer string=w531:string)  [unwired: 1 in]
                n247 = call "Applied Send Command.vi"("error in (no error)"=w527, "Extra"=w531, "Command"=T1."Distance or Position", "VISA resource name"=w526) -> ("error out"=w530:errorcluster, "VISA resource name out"=w525:refnum<visa-resource-name>)  [unwired: 3 in, 1 out]
                n248 = call "Time Delay7"("error in (no error)"=w530, "Delay Time (s)"=w524) -> ("error out"=w528:errorcluster)  [unwired: 9 in]
              }
              frame #2 {
                # "Feed to Position"
                n249 = call "Applied Send Command.vi"("error in (no error)"=w538, "Command"=T1."Feed to Length", "VISA resource name"=w539) -> ("error out"=w533:errorcluster, "VISA resource name out"=w537:refnum<visa-resource-name>)  [unwired: 4 in, 1 out]
                n250 = call "Time Delay5"("error in (no error)"=w533, "Delay Time (s)"=w535) -> ("error out"=w536:errorcluster)  [unwired: 9 in]
              }
            }
            n251 = Decrement(x=w502) -> (x-1=w501:i8)
            n252 = local write "FX Jog counts"(w501) -> ()
            n253 = local write "Jog X-"(FALSE ("Jog X-")) -> ()
          }
        }
      }
      frame #5 {
        n254 = local read "FY Jog Counts In Range?"() -> (w541:bool)
        n255 = local read "Jog Y+"() -> (w540:bool)
        n256 = And(x=w541, y=w540) -> (x .and. y?=w542:bool)
        n257 = case shown="True" w542 {
          tunnel: w544 -> [_ w549]
          tunnel: w543 -> [_ w548]
          frame False {
          }
          frame True {
            n258 = local read "FY Jog counts"() -> (w547:i8)
            n259 = local write "Jog Y+"(FALSE ("Jog Y+")) -> ()
            n260 = Increment(x=w547) -> (x+1=w546:i8)
            n261 = local write "FY Jog counts"(w546) -> ()
            n262 = flat-sequence {
              tunnel: [w562] -> w555
              tunnel: [w557] -> w554
              tunnel: [w556] -> w553
              tunnel: w548 -> [w561]
              tunnel: w549 -> [w560]
              tunnel: [w573] -> w552
              tunnel: [w568] -> w551
              tunnel: w555 -> [w571]
              tunnel: w554 -> [w572]
              tunnel: w553 -> [w569]
              tunnel: [w569] -> w550
              tunnel: [w578] -> _
              tunnel: [w581] -> _
              tunnel: w552 -> [w580]
              tunnel: w551 -> [w579]
              tunnel: w550 -> [w582]
              frame #0 {
                w556 = 0.5 ("Delay Time (s)")
                # "Velocity Setting"
                n263 = property on="Y Velocity SP step/sec" class="DigNum (strict)"() -> ("Value"=w565:i32)  [unwired: 2 in, 2 out]
                n264 = property on="Y steps/rev" class="DigNum (strict)"() -> ("Value"=w564:u32)  [unwired: 2 in, 2 out]
                n265 = Number To Decimal String(number=w565) -> ()  [unwired: 1 in, 1 out]
                n266 = Divide(x=w565, y=w564) -> (x/y=w566:dbl)
                n267 = Number To Fractional String(number=w566) -> (F-format string=w559:string)  [unwired: 3 in]
                n268 = call "Applied Send Command.vi"("error in (no error)"=w561, "Extra"=w559, "Command"=T1."Velocity Setting", "VISA resource name"=w560) -> ("error out"=w558:errorcluster, "VISA resource name out"=w562:refnum<visa-resource-name>)  [unwired: 3 in, 1 out]
                n269 = call "Time Delay22"("error in (no error)"=w558, "Delay Time (s)"=w556) -> ("error out"=w557:errorcluster)  [unwired: 9 in]
              }
              frame #1 {
                # "Move to Abs Position"
                n270 = property on="Y Step SP" class="DigNum (strict)"() -> ("Value"=w575:i32)  [unwired: 2 in, 2 out]
                n271 = Number To Decimal String(number=w575) -> (decimal integer string=w570:string)  [unwired: 1 in]
                n272 = call "Applied Send Command.vi"("error in (no error)"=w572, "Extra"=w570, "Command"=T1."Distance or Position", "VISA resource name"=w571) -> ("error out"=w567:errorcluster, "VISA resource name out"=w573:refnum<visa-resource-name>)  [unwired: 3 in, 1 out]
                n273 = call "Time Delay"("error in (no error)"=w567, "Delay Time (s)"=w569) -> ("error out"=w568:errorcluster)  [unwired: 9 in]
              }
              frame #2 {
                n274 = call "Applied Send Command.vi"("error in (no error)"=w579, "Command"=T1."Feed to Length", "VISA resource name"=w580) -> ("error out"=w576:errorcluster, "VISA resource name out"=w581:refnum<visa-resource-name>)  [unwired: 4 in, 1 out]
                n275 = call "Time Delay23"("error in (no error)"=w576, "Delay Time (s)"=w582) -> ("error out"=w578:errorcluster)  [unwired: 9 in]
              }
            }
          }
        }
      }
      frame #6 {
        n276 = local read "FY Jog Counts In Range?"() -> (w584:bool)
        n277 = local read "Jog Y-"() -> (w583:bool)
        n278 = And(x=w583, y=w584) -> (x .and. y?=w585:bool)
        n279 = case shown="True" w585 {
          tunnel: w587 -> [_ w592]
          tunnel: w586 -> [_ w591]
          frame False {
          }
          frame True {
            n280 = local read "FY Jog counts"() -> (w590:i8)
            n281 = flat-sequence {
              tunnel: [w605] -> w598
              tunnel: [w600] -> w597
              tunnel: [w599] -> w596
              tunnel: w591 -> [w604]
              tunnel: w592 -> [w603]
              tunnel: [w618] -> w595
              tunnel: [w613] -> w594
              tunnel: w598 -> [w616]
              tunnel: w597 -> [w617]
              tunnel: w596 -> [w614]
              tunnel: [w614] -> w593
              tunnel: [w623] -> _
              tunnel: [w626] -> _
              tunnel: w595 -> [w625]
              tunnel: w594 -> [w624]
              tunnel: w593 -> [w627]
              frame #0 {
                w599 = 0.5 ("Delay Time (s)")
                # "Velocity Setting"
                n282 = property on="Y Velocity SP step/sec" class="DigNum (strict)"() -> ("Value"=w608:i32)  [unwired: 2 in, 2 out]
                n283 = property on="Y steps/rev" class="DigNum (strict)"() -> ("Value"=w607:u32)  [unwired: 2 in, 2 out]
                n284 = Number To Decimal String(number=w608) -> ()  [unwired: 1 in, 1 out]
                n285 = Divide(x=w608, y=w607) -> (x/y=w609:dbl)
                n286 = Number To Fractional String(number=w609) -> (F-format string=w602:string)  [unwired: 3 in]
                n287 = call "Applied Send Command.vi"("error in (no error)"=w604, "Extra"=w602, "Command"=T1."Velocity Setting", "VISA resource name"=w603) -> ("error out"=w601:errorcluster, "VISA resource name out"=w605:refnum<visa-resource-name>)  [unwired: 3 in, 1 out]
                n288 = call "Time Delay18"("error in (no error)"=w601, "Delay Time (s)"=w599) -> ("error out"=w600:errorcluster)  [unwired: 9 in]
              }
              frame #1 {
                # "Move to Abs Position"
                n289 = property on="Y Step SP" class="DigNum (strict)"() -> ("Value"=w620:i32)  [unwired: 2 in, 2 out]
                n290 = Multiply(x=-1, y=w620) -> (x*y=w611:i32)
                n291 = Number To Decimal String(number=w611) -> (decimal integer string=w615:string)  [unwired: 1 in]
                n292 = call "Applied Send Command.vi"("error in (no error)"=w617, "Extra"=w615, "Command"=T1."Distance or Position", "VISA resource name"=w616) -> ("error out"=w612:errorcluster, "VISA resource name out"=w618:refnum<visa-resource-name>)  [unwired: 3 in, 1 out]
                n293 = call "Time Delay10"("error in (no error)"=w612, "Delay Time (s)"=w614) -> ("error out"=w613:errorcluster)  [unwired: 9 in]
              }
              frame #2 {
                n294 = call "Applied Send Command.vi"("error in (no error)"=w624, "Command"=T1."Feed to Length", "VISA resource name"=w625) -> ("error out"=w621:errorcluster, "VISA resource name out"=w626:refnum<visa-resource-name>)  [unwired: 4 in, 1 out]
                n295 = call "Time Delay9"("error in (no error)"=w621, "Delay Time (s)"=w627) -> ("error out"=w623:errorcluster)  [unwired: 9 in]
              }
            }
            n296 = Decrement(x=w590) -> (x-1=w589:i8)
            n297 = local write "FY Jog counts"(w589) -> ()
            n298 = local write "Jog Y-"(FALSE ("Jog Y-")) -> ()
          }
        }
      }
      frame #7 {
        n299 = local read "FZ Jog Counts In Range?"() -> (w629:bool)
        n300 = local read "Jog Z+"() -> (w628:bool)
        n301 = And(x=w628, y=w629) -> (x .and. y?=w630:bool)
        n302 = case shown="True" w630 {
          tunnel: w632 -> [_ w637]
          tunnel: w631 -> [_ w636]
          frame False {
          }
          frame True {
            n303 = local read "FZ Jog counts"() -> (w635:i8)
            n304 = flat-sequence {
              tunnel: [w649] -> w643
              tunnel: [w647] -> w642
              tunnel: [w646] -> w641
              tunnel: w637 -> [w645]
              tunnel: w636 -> [w644]
              tunnel: [w658] -> w640
              tunnel: [w657] -> w639
              tunnel: w643 -> [w659]
              tunnel: w642 -> [w661]
              tunnel: w641 -> [w655]
              tunnel: [w655] -> w638
              tunnel: [w670] -> _
              tunnel: [w667] -> _
              tunnel: w640 -> [w668]
              tunnel: w639 -> [w666]
              tunnel: w638 -> [w669]
              frame #0 {
                w646 = 0.1 ("Delay Time (s)")
                n305 = property on="Z Velocity SP step/sec" class="DigNum (strict)"() -> ("Value"=w651:i32)  [unwired: 2 in, 2 out]
                n306 = property on="Z steps/rev" class="DigNum (strict)"() -> ("Value"=w650:u32)  [unwired: 2 in, 2 out]
                n307 = Divide(x=w651, y=w650) -> (x/y=w652:dbl)
                n308 = Number To Fractional String(number=w652) -> (F-format string=w653:string)  [unwired: 3 in]
                n309 = call "Applied Send Command.vi"("error in (no error)"=w644, "Extra"=w653, "Command"=T1."Velocity Setting", "VISA resource name"=w645) -> ("error out"=w648:errorcluster, "VISA resource name out"=w649:refnum<visa-resource-name>)  [unwired: 3 in, 1 out]
                n310 = call "Time Delay52"("error in (no error)"=w648, "Delay Time (s)"=w646) -> ("error out"=w647:errorcluster)  [unwired: 9 in]
              }
              frame #1 {
                # "Move to Abs Position"
                n311 = property on="Z Step SP" class="DigNum (strict)"() -> ("Value"=w663:i32)  [unwired: 2 in, 2 out]
                n312 = Number To Decimal String(number=w663) -> (decimal integer string=w660:string)  [unwired: 1 in]
                n313 = call "Applied Send Command.vi"("error in (no error)"=w661, "Extra"=w660, "Command"=T1."Distance or Position", "VISA resource name"=w659) -> ("error out"=w656:errorcluster, "VISA resource name out"=w658:refnum<visa-resource-name>)  [unwired: 3 in, 1 out]
                n314 = call "Time Delay51"("error in (no error)"=w656, "Delay Time (s)"=w655) -> ("error out"=w657:errorcluster)  [unwired: 9 in]
              }
              frame #2 {
                n315 = call "Applied Send Command.vi"("error in (no error)"=w666, "Command"=T1."Feed to Length", "VISA resource name"=w668) -> ("error out"=w664:errorcluster, "VISA resource name out"=w667:refnum<visa-resource-name>)  [unwired: 4 in, 1 out]
                n316 = call "Time Delay28"("error in (no error)"=w664, "Delay Time (s)"=w669) -> ("error out"=w670:errorcluster)  [unwired: 9 in]
              }
            }
            n317 = Increment(x=w635) -> (x+1=w634:i8)
            n318 = local write "FZ Jog counts"(w634) -> ()
            n319 = local write "Jog Z+"(FALSE ("Jog Z+")) -> ()
          }
        }
      }
      frame #8 {
        n320 = local read "Jog Z-"() -> (w671:bool)
        n321 = local read "FZ Jog Counts In Range?"() -> (w672:bool)
        n322 = And(x=w672, y=w671) -> (x .and. y?=w673:bool)
        n323 = case shown="True" w673 {
          tunnel: w675 -> [_ w680]
          tunnel: w674 -> [_ w679]
          frame False {
          }
          frame True {
            n324 = local read "FZ Jog counts"() -> (w678:i8)
            n325 = flat-sequence {
              tunnel: [w690] -> w686
              tunnel: [w688] -> w685
              tunnel: [w687] -> w684
              tunnel: w679 -> [w691]
              tunnel: w680 -> [w692]
              tunnel: [w703] -> w683
              tunnel: [w702] -> w682
              tunnel: w686 -> [w704]
              tunnel: w685 -> [w706]
              tunnel: w684 -> [w700]
              tunnel: [w700] -> w681
              tunnel: [w715] -> _
              tunnel: [w712] -> _
              tunnel: w683 -> [w713]
              tunnel: w682 -> [w711]
              tunnel: w681 -> [w714]
              frame #0 {
                w687 = 0.1 ("Delay Time (s)")
                n326 = property on="Z Velocity SP step/sec" class="DigNum (strict)"() -> ("Value"=w694:i32)  [unwired: 2 in, 2 out]
                n327 = property on="Z steps/rev" class="DigNum (strict)"() -> ("Value"=w693:u32)  [unwired: 2 in, 2 out]
                n328 = Divide(x=w694, y=w693) -> (x/y=w695:dbl)
                n329 = Number To Fractional String(number=w695) -> (F-format string=w696:string)  [unwired: 3 in]
                n330 = call "Applied Send Command.vi"("error in (no error)"=w691, "Extra"=w696, "Command"=T1."Velocity Setting", "VISA resource name"=w692) -> ("error out"=w689:errorcluster, "VISA resource name out"=w690:refnum<visa-resource-name>)  [unwired: 3 in, 1 out]
                n331 = call "Time Delay21"("error in (no error)"=w689, "Delay Time (s)"=w687) -> ("error out"=w688:errorcluster)  [unwired: 9 in]
              }
              frame #1 {
                # "Move to Abs Position"
                n332 = property on="Z Step SP" class="DigNum (strict)"() -> ("Value"=w708:i32)  [unwired: 2 in, 2 out]
                n333 = Multiply(x=-1, y=w708) -> (x*y=w699:i32)
                n334 = Number To Decimal String(number=w699) -> (decimal integer string=w705:string)  [unwired: 1 in]
                n335 = call "Applied Send Command.vi"("error in (no error)"=w706, "Extra"=w705, "Command"=T1."Distance or Position", "VISA resource name"=w704) -> ("error out"=w701:errorcluster, "VISA resource name out"=w703:refnum<visa-resource-name>)  [unwired: 3 in, 1 out]
                n336 = call "Time Delay20"("error in (no error)"=w701, "Delay Time (s)"=w700) -> ("error out"=w702:errorcluster)  [unwired: 9 in]
              }
              frame #2 {
                n337 = call "Applied Send Command.vi"("error in (no error)"=w711, "Command"=T1."Feed to Length", "VISA resource name"=w713) -> ("error out"=w709:errorcluster, "VISA resource name out"=w712:refnum<visa-resource-name>)  [unwired: 4 in, 1 out]
                n338 = call "Time Delay19"("error in (no error)"=w709, "Delay Time (s)"=w714) -> ("error out"=w715:errorcluster)  [unwired: 9 in]
              }
            }
            n339 = Decrement(x=w678) -> (x-1=w677:i8)
            n340 = local write "FZ Jog counts"(w677) -> ()
            n341 = local write "Jog Z-"(FALSE ("Jog Z-")) -> ()
          }
        }
      }
      frame #9 {
        n342 = local read "Movex4Z REQ"() -> (w717:bool)
        n343 = And(x=FALSE, y=w717) -> (x .and. y?=w716:bool)
        n344 = case shown="True" w716 {
          tunnel: w719 -> [_ w724]
          tunnel: w720 -> [_ w723]
          frame False {
          }
          frame True {
            n345 = flat-sequence {
              tunnel: [w736] -> w730
              tunnel: [w734] -> w729
              tunnel: [w733] -> w728
              tunnel: w724 -> [w732]
              tunnel: w723 -> [w731]
              tunnel: [w748] -> w727
              tunnel: [w747] -> w726
              tunnel: w730 -> [w749]
              tunnel: w729 -> [w751]
              tunnel: w728 -> [w745]
              tunnel: [w745] -> w725
              tunnel: [w759] -> _
              tunnel: [w756] -> _
              tunnel: w727 -> [w757]
              tunnel: w726 -> [w755]
              tunnel: w725 -> [w758]
              frame #0 {
                w733 = 0.1 ("Delay Time (s)")
                n346 = property on="Z  velocity PV step/sec" class="DigNum (strict)"() -> ("Value"=w738:i32)  [unwired: 2 in, 2 out]
                n347 = property on="Z steps/rev" class="DigNum (strict)"() -> ("Value"=w737:u32)  [unwired: 2 in, 2 out]
                n348 = Divide(x=w738, y=w737) -> (x/y=w739:dbl)
                n349 = Number To Fractional String(number=w739) -> (F-format string=w740:string)  [unwired: 3 in]
                n350 = call "Applied Send Command.vi"("error in (no error)"=w731, "Extra"=w740, "Command"=T1."Velocity Setting", "VISA resource name"=w732) -> ("error out"=w735:errorcluster, "VISA resource name out"=w736:refnum<visa-resource-name>)  [unwired: 3 in, 1 out]
                n351 = call "Time Delay24"("error in (no error)"=w735, "Delay Time (s)"=w733) -> ("error out"=w734:errorcluster)  [unwired: 9 in]
              }
              frame #1 {
                # "Move to Abs Position"
                n352 = property on="Z Step SP" class="DigNum (strict)"() -> ("Value"=w744:i32)  [unwired: 2 in, 2 out]
                n353 = Multiply(x=w744, y=1) -> (x*y=w742:i32)
                n354 = Number To Decimal String(number=w742) -> (decimal integer string=w750:string)  [unwired: 1 in]
                n355 = call "Applied Send Command.vi"("error in (no error)"=w751, "Extra"=w750, "Command"=T1."Distance or Position", "VISA resource name"=w749) -> ("error out"=w746:errorcluster, "VISA resource name out"=w748:refnum<visa-resource-name>)  [unwired: 3 in, 1 out]
                n356 = call "Time Delay25"("error in (no error)"=w746, "Delay Time (s)"=w745) -> ("error out"=w747:errorcluster)  [unwired: 9 in]
              }
              frame #2 {
                n357 = call "Applied Send Command.vi"("error in (no error)"=w755, "Command"=T1."Feed to Length", "VISA resource name"=w757) -> ("error out"=w753:errorcluster, "VISA resource name out"=w756:refnum<visa-resource-name>)  [unwired: 4 in, 1 out]
                n358 = call "Time Delay26"("error in (no error)"=w753, "Delay Time (s)"=w758) -> ("error out"=w759:errorcluster)  [unwired: 9 in]
              }
            }
            n359 = local write "FZ Jog counts"(i8 0 ("FZ Jog counts")) -> ()
            n360 = local write "Movex4Z REQ"(FALSE ("Move 5Z REQ")) -> ()
          }
        }
      }
    }
    n361 = flat-sequence {
      frame #0 {
      }
    }
    n362 = flat-sequence {
      frame #0 {
        w308 = 0 ("index (col)")
        w361 = 0.0 ("element")
        n363 = Build Array("APX:FX_UP", "APX:FX_DOWN", "APX:FY_UP", "APX:FY_DOWN", "APX:FZ_UP", "APX:FZ_DOWN", "APX:FZ_UPUP", "APX:FZ_DOWNDOWN") -> (w321:string[])
        n364 = call-poly "CaLabGet.vi"("PV Names"=w321) -> ("Value Array (number)"=w309:dbl[][])  [unwired: 8 in, 6 out]
        n365 = Reshape Array(w309, 6 ("dimension size")) -> (w317:dbl[])
        n366 = Add Array Elements(numeric array=w317) -> (sum=w323:dbl)
        n367 = Build Array(w361, w361, w361, w361, w361, w361) -> (w320:dbl[])
        n368 = Not Equal?(x=w323, y=0.0) -> (x != y?=w319:bool)
        n369 = case shown="True" w319 {
          tunnel: w321 -> [_ w369]
          tunnel: w320 -> [_ w368]
          frame False {
          }
          frame True {
            n370 = call-poly <userlib>:"CaLabPut.vi"("Values"=w368, "PV Names"=w369) -> ()  [unwired: 6 in, 4 out]
          }
        }
        n371 = Index Array(array=w309, index (row)=0 ("disabled index (row)"), index (col)=w308) -> (element=w348:dbl)
        "APX:FX_UP" <- w348
        n372 = Index Array(array=w309, index (row)=1, index (col)=w308) -> (element=w347:dbl)
        "APX:FX_DOWN" <- w347
        n373 = Index Array(array=w309, index (row)=4, index (col)=w308) -> (element=w315:dbl)
        "APX:FZ_UP" <- w315
        n374 = Index Array(array=w309, index (row)=2, index (col)=w308) -> (element=w346:dbl)
        "APX:FY_UP" <- w346
        n375 = Index Array(array=w309, index (row)=5, index (col)=w308) -> (element=w344:dbl)
        "APX:FZ_DOWN" <- w344
        n376 = Index Array(array=w309, index (row)=3, index (col)=w308) -> (element=w345:dbl)
        "APX:FY_DOWN" <- w345
        n377 = Index Array(array=w309, index (row)=6 ("disabled index (row)"), index (col)=w308) -> (element=w305:dbl)
        n378 = Index Array(array=w309, index (row)=7 ("disabled index (row)"), index (col)=w308) -> (element=w301:dbl)
        n379 = Number To Boolean Array(number=w348) -> (Boolean array=w343:bool[])
        n380 = Number To Boolean Array(number=w347) -> (Boolean array=w341:bool[])
        n381 = Number To Boolean Array(number=w346) -> (Boolean array=w339:bool[])
        n382 = Number To Boolean Array(number=w315) -> (Boolean array=w335:bool[])
        n383 = Number To Boolean Array(number=w344) -> (Boolean array=w333:bool[])
        n384 = Number To Boolean Array(number=w301) -> (Boolean array=w300:bool[])
        n385 = Number To Boolean Array(number=w345) -> (Boolean array=w337:bool[])
        n386 = Number To Boolean Array(number=w305) -> (Boolean array=w304:bool[])
        n387 = Index Array(array=w343, index=0) -> (element=w331:bool)
        n388 = Index Array(array=w341, index=0) -> (element=w330:bool)
        n389 = Index Array(array=w337, index=0) -> (element=w328:bool)
        n390 = Index Array(array=w339, index=0) -> (element=w329:bool)
        n391 = Index Array(array=w335, index=0) -> (element=w327:bool)
        n392 = Index Array(array=w300, index=0) -> (element=w298:bool)
        n393 = Index Array(array=w333, index=0) -> (element=w326:bool)
        n394 = Index Array(array=w304, index=0) -> (element=w302:bool)
        n395 = Scale By Power Of 2(n=w315, x=0.5) -> (x*2^n=→"x*2^n":dbl)
        n396 = case shown="False" "Local" {
          tunnel: [w372 "Jog Z- CNTL"] -> w354
          tunnel: [w373 "Jog Z+ CNTL"] -> w353
          tunnel: [w374 "Jog Y- CNTL"] -> w352
          tunnel: [w375 "Jog Y+ CNTL"] -> w351
          tunnel: [w376 "Jog X- CNTL"] -> w350
          tunnel: [w377 "Jog X+ CNTL"] -> w349
          tunnel: w331 -> [w377 _]
          tunnel: w330 -> [w376 _]
          tunnel: w329 -> [w375 _]
          tunnel: w328 -> [w374 _]
          tunnel: w327 -> [w373 _]
          tunnel: w326 -> [w372 _]
          tunnel: w321 -> [_ _]
          tunnel: w320 -> [_ _]
          tunnel: [w371 "Jog Z++ CNTL"] -> w311
          tunnel: [w370 "Jog Z-- CNTL"] -> w310
          tunnel: w302 -> [w371 _]
          tunnel: w298 -> [w370 _]
          frame False {
          }
          frame True {
          }
        }
        "Jog X+" <- w349
        "Jog X-" <- w350
        "Jog Y+" <- w351
        "Jog Y-" <- w352
        "Jog Z+" <- w353
        "Jog Z-" <- w354
        "Jog Z4+" <- w311
        "Jog Z4-" <- w310
        "Movex4Z REQ" <- "Move x4Z"
      }
    }
    n397 = event shown="[1] \"Reset Y Position mm\", \"Reset X Position mm\", \"Reset Z Position mm\": Value Change" {
      selector: _ -> [_ _ _ _ _ _]
      dyn-events: _ -> [_ _ _ _ _ _]
      timeout: 1 -> [_ _ _ _ _ _]
      tunnel: w275 -> [w840 _ _ w1078 w1090 w1117]
      tunnel: [_ _ _ w1078 w1088 w1115] -> w296
      tunnel: w276 -> [w812 _ _ w1079 w1091 w1118]
      tunnel: [_ _ _ w1079 w1089 w1116] -> w295
      tunnel: w278 -> [w811 _ _ _ w1085 w1114]
      tunnel: w277 -> [w823 _ _ _ w1084 w1113]
      tunnel: [_ _ _ _ w1087 w1112] -> w293
      tunnel: [_ _ _ _ w1086 w1111] -> w292
      tunnel: w274 -> [w813 _ _ _ w1083 w1110]
      tunnel: w273 -> [w814 _ _ _ w1082 w1109]
      tunnel: [_ _ _ _ w1081 _] -> w291
      tunnel: [_ _ _ _ w1080 _] -> w290
      tunnel: [_ _ _ _ _ w1108] -> w289
      tunnel: [_ _ _ _ _ w1107] -> w288
      event Timeout {
        n398 = event-data() -> ()  [unwired: 1 in, 2 out]
        n399 = flat-sequence {
          tunnel: [w852] -> w822
          tunnel: [w865] -> w821
          tunnel: [w874] -> w820
          tunnel: [w845] -> w819
          tunnel: w813 -> [w860]
          tunnel: w814 -> [w861]
          tunnel: [w843] -> w780
          tunnel: w822 -> [w884]
          tunnel: [w884] -> w818
          tunnel: w821 -> [w883]
          tunnel: [w883] -> w817
          tunnel: w820 -> [w882]
          tunnel: [w879] -> w816
          tunnel: w819 -> [w881]
          tunnel: [w881] -> w815
          tunnel: w818 -> [w887]
          tunnel: w817 -> [w888]
          tunnel: w816 -> [w886]
          tunnel: w815 -> [w885]
          tunnel: [w885] -> w788
          frame #0 {
            w864 = 0.5 ("Delay Time (s)")
            n400 = call "Applied Send Command.vi"("error in (no error)"=w861, "Command"=T1."Immediate Position?", "VISA resource name"=w860) -> ("error out"=w859:errorcluster, "read buffer"=w856:string, "VISA resource name out"=w854:refnum<visa-resource-name>)  [unwired: 4 in]
            n401 = Hexadecimal String To Number(string=w856, offset=3) -> (number=w857:u32)  [unwired: 1 in, 1 out]
            n402 = property on="Z Step SP" class="DigNum (strict)"() -> ("Maximum"=w876:dbl)  [unwired: 2 in, 2 out]
            n403 = property on="Z Step SP" class="DigNum (strict)"() -> ("Minimum"=w878:dbl)  [unwired: 2 in, 2 out]
            n404 = To Long Integer(number=w857) -> (32bit integer=w866:i32)
            n405 = property on="Z steps/rev" class="DigNum (strict)"() -> ("Value"=w872:u32)  [unwired: 2 in, 2 out]
            n406 = property on="Z Step PV" class="DigNum (strict)"("Val(Sgnl)"=w866) -> ()  [unwired: 2 in, 2 out]
            n407 = To Long Integer(number=w876) -> (32bit integer=w875:i32)
            n408 = To Long Integer(number=w878) -> (32bit integer=w877:i32)
            n409 = In Range and Coerce(upper limit=w875, x=w866, lower limit=w877) -> (In Range?=w874:bool)  [unwired: 1 out]
            n410 = To Double Precision Float(number=w866) -> (double precision float=w867:dbl)
            n411 = To Double Precision Float(number=w872) -> (double precision float=w873:dbl)
            n412 = property on="Z in Range" class="Bool (strict)"("Val(Sgnl)"=w874) -> ()  [unwired: 2 in, 2 out]
            n413 = Divide(x=w867, y=w873) -> (x/y=w871:dbl)
            n414 = call "Time Delay17"("error in (no error)"=w859, "Delay Time (s)"=w864) -> ("error out"=w844:errorcluster)  [unwired: 9 in]
            n415 = property on="Z mm/rev" class="DigNum (strict)"() -> ("Value"=w870:dbl)  [unwired: 2 in, 2 out]
            n416 = property on="Z offset mm" class="DigNum (strict)"() -> ("Value"=w868:dbl)  [unwired: 2 in, 2 out]
            n417 = Multiply(x=w871, y=w870) -> (x*y=w869:dbl)
            n418 = call "Applied Send Command.vi"("error in (no error)"=w844, "Command"=T1."Request Status", "VISA resource name"=w854) -> ("error out"=w853:errorcluster, "read buffer"=w849:string, "VISA resource name out"=w852:refnum<visa-resource-name>)  [unwired: 4 in]
            n419 = call "Time Delay16"("error in (no error)"=w853, "Delay Time (s)"=w864) -> ("error out"=w865:errorcluster)  [unwired: 9 in]
            n420 = Add(x=w869, y=w868) -> (x+y=w843:dbl)
            n421 = String Subset(string=w849, offset (0)=0, length (rest)=1 ("length (rest)")) -> (substring=w846:string)
            n422 = property on="Z Position mm PV" class="DigNum (strict)"("Val(Sgnl)"=w843) -> ()  [unwired: 2 in, 2 out]
            n423 = Equal?(x=w846, y="R") -> (x = y?=w863:bool)
            n424 = Not Equal?(x=w846, y="R") -> (x != y?=w845:bool)
            n425 = property on="Z Ready" class="Bool (strict)"("Val(Sgnl)"=w863) -> ()  [unwired: 2 in, 2 out]
            n426 = property on="Z in Motion" class="Bool (strict)"("Val(Sgnl)"=w845) -> ()  [unwired: 2 in, 2 out]
          }
          frame #1 {
            n427 = local read "Isolated from GND?"() -> (w880:bool)
            n428 = Or(x=w880, y=w882) -> (x .or. y?=w879:bool)
          }
          frame #2 {
            n429 = case shown="False" w886 {
              tunnel: w887 -> [w892 w895]
              tunnel: [w890 w895] -> _
              tunnel: [w889 w894] -> _
              tunnel: w888 -> [w891 w894]
              frame False {
                n430 = call "Applied Send Command.vi"("error in (no error)"=w891, "Command"=T1."Stop & Kill Buffer", "VISA resource name"=w892) -> ("error out"=w889:errorcluster, "VISA resource name out"=w890:refnum<visa-resource-name>)  [unwired: 4 in, 1 out]
              }
              frame True {
              }
            }
          }
        }
        n431 = property on="Y Step SP" class="DigNum (strict)"() -> ("Maximum"=w808:dbl)  [unwired: 2 in, 2 out]
        n432 = property on="Y Step SP" class="DigNum (strict)"() -> ("Minimum"=w807:dbl)  [unwired: 2 in, 2 out]
        n433 = property on="X Step SP" class="DigNum (strict)"() -> ("Maximum"=w803:dbl)  [unwired: 2 in, 2 out]
        n434 = property on="X Step SP" class="DigNum (strict)"() -> ("Minimum"=w804:dbl)  [unwired: 2 in, 2 out]
        n435 = Subtract(x=w808, y=w807) -> (x-y=w809:dbl)
        n436 = Subtract(x=w803, y=w804) -> (x-y=w805:dbl)
        n437 = property on="X Step PV" class="DigNum (strict)"() -> ("Value"=w802:i32)  [unwired: 2 in, 2 out]
        n438 = property on="Y Step PV" class="DigNum (strict)"() -> ("Value"=w801:i32)  [unwired: 2 in, 2 out]
        n439 = Divide(x=w809, y=2.0) -> (x/y=w797:dbl)
        n440 = Divide(x=w805, y=2.0) -> (x/y=w798:dbl)
        n441 = Absolute Value(x=w802) -> (abs(x)=w799:i32)
        n442 = Absolute Value(x=w801) -> (abs(x)=w800:i32)
        n443 = Absolute Value(x=w797) -> (abs(x)=w795:dbl)
        n444 = Absolute Value(x=w798) -> (abs(x)=w796:dbl)
        n445 = Multiply(x=w799, y=w800) -> (x*y=w794:i32)
        n446 = Multiply(x=w795, y=w796) -> (x*y=w793:dbl)
        n447 = Less Or Equal?(x=w794, y=w793) -> (x <= y?=w792:bool)
        n448 = flat-sequence {
          tunnel: w840 -> [w968]
          tunnel: w812 -> [w969]
          tunnel: [w965] -> w839
          tunnel: [w975] -> w837
          tunnel: [w954] -> w835
          tunnel: [w956] -> w833
          tunnel: w808 -> [w955]
          tunnel: w807 -> [w952]
          tunnel: w792 -> [w953]
          tunnel: [w951] -> w781
          tunnel: w839 -> [w994]
          tunnel: [w994] -> w838
          tunnel: w837 -> [w993]
          tunnel: [w993] -> w836
          tunnel: w835 -> [w992]
          tunnel: [w990] -> w834
          tunnel: w833 -> [w991]
          tunnel: [w991] -> w832
          tunnel: w838 -> [w997]
          tunnel: w836 -> [w998]
          tunnel: w834 -> [w996]
          tunnel: w832 -> [w995]
          tunnel: [w995] -> w789
          frame #0 {
            w974 = 0.5 ("Delay Time (s)")
            n449 = call "Applied Send Command.vi"("error in (no error)"=w968, "Command"=T1."Immediate Position?", "VISA resource name"=w969) -> ("error out"=w971:errorcluster, "read buffer"=w972:string, "VISA resource name out"=w966:refnum<visa-resource-name>)  [unwired: 4 in]
            n450 = To Long Integer(number=w955) -> (32bit integer=w986:i32)
            n451 = To Long Integer(number=w952) -> (32bit integer=w987:i32)
            n452 = Hexadecimal String To Number(string=w972, offset=3) -> (number=w976:u32)  [unwired: 1 in, 1 out]
            n453 = To Long Integer(number=w976) -> (32bit integer=w977:i32)
            n454 = property on="Y steps/rev" class="DigNum (strict)"() -> ("Value"=w983:u32)  [unwired: 2 in, 2 out]
            n455 = property on="Y Step PV" class="DigNum (strict)"("Val(Sgnl)"=w977) -> ()  [unwired: 2 in, 2 out]
            n456 = In Range and Coerce(upper limit=w986, x=w977, lower limit=w987) -> (In Range?=w985:bool)  [unwired: 1 out]
            n457 = To Double Precision Float(number=w977) -> (double precision float=w978:dbl)
            n458 = To Double Precision Float(number=w983) -> (double precision float=w984:dbl)
            n459 = Divide(x=w978, y=w984) -> (x/y=w982:dbl)
            n460 = And(x=w985, y=w953) -> (x .and. y?=w954:bool)
            n461 = property on="Y in Range" class="Bool (strict)"("Val(Sgnl)"=w954) -> ()  [unwired: 2 in, 2 out]
            n462 = call "Time Delay4"("error in (no error)"=w971, "Delay Time (s)"=w974) -> ("error out"=w964:errorcluster)  [unwired: 9 in]
            n463 = property on="Y mm/rev" class="DigNum (strict)"() -> ("Value"=w981:dbl)  [unwired: 2 in, 2 out]
            n464 = property on="Y offset mm" class="DigNum (strict)"() -> ("Value"=w979:dbl)  [unwired: 2 in, 2 out]
            n465 = Multiply(x=w982, y=w981) -> (x*y=w980:dbl)
            n466 = call "Applied Send Command.vi"("error in (no error)"=w964, "Command"=T1."Request Status", "VISA resource name"=w966) -> ("error out"=w963:errorcluster, "read buffer"=w960:string, "VISA resource name out"=w965:refnum<visa-resource-name>)  [unwired: 4 in]
            n467 = call "Time Delay3"("error in (no error)"=w963, "Delay Time (s)"=w974) -> ("error out"=w975:errorcluster)  [unwired: 9 in]
            n468 = Add(x=w980, y=w979) -> (x+y=w951:dbl)
            n469 = String Subset(string=w960, offset (0)=0, length (rest)=1 ("length (rest)")) -> (substring=w958:string)
            n470 = property on="Y Position mm PV" class="DigNum (strict)"("Val(Sgnl)"=w951) -> ()  [unwired: 2 in, 2 out]
            n471 = Equal?(x=w958, y="R") -> (x = y?=w973:bool)
            n472 = Not Equal?(x=w958, y="R") -> (x != y?=w956:bool)
            n473 = property on="Y Ready" class="Bool (strict)"("Val(Sgnl)"=w973) -> ()  [unwired: 2 in, 2 out]
            n474 = property on="Y in Motion" class="Bool (strict)"("Val(Sgnl)"=w956) -> ()  [unwired: 2 in, 2 out]
          }
          frame #1 {
            n475 = local read "Isolated from GND?"() -> (w989:bool)
            n476 = Or(x=w992, y=w989) -> (x .or. y?=w990:bool)
          }
          frame #2 {
            n477 = case shown="False" w996 {
              tunnel: w997 -> [w1000 w1005]
              tunnel: [w1002 w1005] -> _
              tunnel: [w1001 w1004] -> _
              tunnel: w998 -> [w999 w1004]
              frame False {
                n478 = call "Applied Send Command.vi"("error in (no error)"=w999, "Command"=T1."Stop & Kill Buffer", "VISA resource name"=w1000) -> ("error out"=w1001:errorcluster, "VISA resource name out"=w1002:refnum<visa-resource-name>)  [unwired: 4 in, 1 out]
              }
              frame True {
              }
            }
          }
        }
        n479 = flat-sequence {
          tunnel: [w909] -> w831
          tunnel: [w920] -> w830
          tunnel: [w898] -> w829
          tunnel: [w905] -> w828
          tunnel: w811 -> [w916]
          tunnel: w823 -> [w904]
          tunnel: w803 -> [w900]
          tunnel: w804 -> [w899]
          tunnel: w792 -> [w897]
          tunnel: [w896] -> w782
          tunnel: w831 -> [w939]
          tunnel: [w939] -> w827
          tunnel: w830 -> [w938]
          tunnel: [w938] -> w826
          tunnel: w829 -> [w935]
          tunnel: [w934] -> w825
          tunnel: w828 -> [w937]
          tunnel: [w937] -> w824
          tunnel: w827 -> [w943]
          tunnel: w826 -> [w942]
          tunnel: w825 -> [w941]
          tunnel: w824 -> [w940]
          tunnel: [w940] -> w790
          frame #0 {
            w919 = 0.5 ("Delay Time (s)")
            n480 = To Long Integer(number=w899) -> (32bit integer=w932:i32)
            n481 = To Long Integer(number=w900) -> (32bit integer=w931:i32)
            n482 = call "Applied Send Command.vi"("error in (no error)"=w904, "Command"=T1."Immediate Position?", "VISA resource name"=w916) -> ("error out"=w914:errorcluster, "read buffer"=w915:string, "VISA resource name out"=w910:refnum<visa-resource-name>)  [unwired: 4 in]
            n483 = Hexadecimal String To Number(string=w915, offset=3) -> (number=w921:u32)  [unwired: 1 in, 1 out]
            n484 = To Long Integer(number=w921) -> (32bit integer=w922:i32)
            n485 = property on="X steps/rev" class="DigNum (strict)"() -> ("Value"=w928:u32)  [unwired: 2 in, 2 out]
            n486 = property on="X Step PV" class="DigNum (strict)"("Val(Sgnl)"=w922) -> ()  [unwired: 2 in, 2 out]
            n487 = In Range and Coerce(upper limit=w931, x=w922, lower limit=w932) -> (In Range?=w930:bool)  [unwired: 1 out]
            n488 = To Double Precision Float(number=w922) -> (double precision float=w923:dbl)
            n489 = To Double Precision Float(number=w928) -> (double precision float=w929:dbl)
            n490 = Divide(x=w923, y=w929) -> (x/y=w927:dbl)
            n491 = And(x=w897, y=w930) -> (x .and. y?=w898:bool)
            n492 = property on="X  in Range" class="Bool (strict)"("Val(Sgnl)"=w898) -> ()  [unwired: 2 in, 2 out]
            n493 = call "Time Delay12"("error in (no error)"=w914, "Delay Time (s)"=w919) -> ("error out"=w907:errorcluster)  [unwired: 9 in]
            n494 = property on="X mm/rev" class="DigNum (strict)"() -> ("Value"=w926:dbl)  [unwired: 2 in, 2 out]
            n495 = property on="X offset mm" class="DigNum (strict)"() -> ("Value"=w924:dbl)  [unwired: 2 in, 2 out]
            n496 = Multiply(x=w927, y=w926) -> (x*y=w925:dbl)
            n497 = call "Applied Send Command.vi"("error in (no error)"=w907, "Command"=T1."Request Status", "VISA resource name"=w910) -> ("error out"=w908:errorcluster, "read buffer"=w912:string, "VISA resource name out"=w909:refnum<visa-resource-name>)  [unwired: 4 in]
            n498 = call "Time Delay11"("error in (no error)"=w908, "Delay Time (s)"=w919) -> ("error out"=w920:errorcluster)  [unwired: 9 in]
            n499 = Add(x=w925, y=w924) -> (x+y=w896:dbl)
            n500 = String Subset(string=w912, offset (0)=0, length (rest)=1 ("length (rest)")) -> (substring=w901:string)
            n501 = property on="X Position mm PV" class="DigNum (strict)"("Val(Sgnl)"=w896) -> ()  [unwired: 2 in, 2 out]
            n502 = Equal?(x=w901, y="R") -> (x = y?=w918:bool)
            n503 = Not Equal?(x=w901, y="R") -> (x != y?=w905:bool)
            n504 = property on="X Ready" class="Bool (strict)"("Val(Sgnl)"=w918) -> ()  [unwired: 2 in, 2 out]
            n505 = property on="X  in Motion" class="Bool (strict)"("Val(Sgnl)"=w905) -> ()  [unwired: 2 in, 2 out]
          }
          frame #1 {
            n506 = local read "Isolated from GND?"() -> (w936:bool)
            n507 = Or(x=w936, y=w935) -> (x .or. y?=w934:bool)
          }
          frame #2 {
            n508 = case shown="False" w941 {
              tunnel: w943 -> [w945 w950]
              tunnel: [w947 w950] -> _
              tunnel: [w948 w949] -> _
              tunnel: w942 -> [w944 w949]
              frame False {
                n509 = call "Applied Send Command.vi"("error in (no error)"=w944, "Command"=T1."Stop & Kill Buffer", "VISA resource name"=w945) -> ("error out"=w948:errorcluster, "VISA resource name out"=w947:refnum<visa-resource-name>)  [unwired: 4 in, 1 out]
              }
              frame True {
              }
            }
          }
        }
        n510 = Compound Arithmetic op=OR(w790, w789, w788) -> (w791:bool)
        n511 = case shown="False" w791 {
          tunnel: [T2."Enabled" ("Disabled") T2."Disabled and Grayed Out" ("Disabled")] -> w787
          frame False {
          }
          frame True {
          }
        }
        n512 = Build Array("APX:PiezoX", "APX:PiezoY", "APX:PiezoZ") -> (w786:string[])
        n513 = Build Array(w782, w781, w780) -> (w779:dbl[])
        n514 = call-poly <userlib>:"CaLabPut.vi"("Values"=w779, "PV Names"=w786) -> ()  [unwired: 6 in, 4 out]
        n515 = property on="Jog X-" class="Bool"("DisabledEnum"=w787) -> ()  [unwired: 2 in, 2 out]
        n516 = property on="Jog X+" class="Bool"("DisabledEnum"=w787) -> ()  [unwired: 2 in, 2 out]
        n517 = property on="Jog Y+" class="Bool"("DisabledEnum"=w787) -> ()  [unwired: 2 in, 2 out]
        n518 = property on="Jog Z+" class="Bool"("DisabledEnum"=w787) -> ()  [unwired: 2 in, 2 out]
        n519 = property on="Jog Y-" class="Bool"("DisabledEnum"=w787) -> ()  [unwired: 2 in, 2 out]
        n520 = property on="Jog Z-" class="Bool"("DisabledEnum"=w787) -> ()  [unwired: 2 in, 2 out]
      }
      event "Reset Y Position mm", "Reset X Position mm", "Reset Z Position mm": Value Change {
        n521 = event-data() -> ()  [unwired: 1 in, 5 out]
        n522 = flat-sequence {
          frame #0 {
            n523 = property on="Reset Y Position mm" class="DigNum (strict)"() -> ("Value"=w1032:dbl)  [unwired: 2 in, 2 out]
            n524 = property on="Reset X Position mm" class="DigNum (strict)"() -> ("Value"=w1023:dbl)  [unwired: 2 in, 2 out]
            n525 = property on="Reset Z Position mm" class="DigNum (strict)"() -> ("Value"=w1014:dbl)  [unwired: 2 in, 2 out]
            n526 = property on="Y offset mm" class="DigNum (strict)"() -> ("Value"=w1024:dbl)  [unwired: 2 in, 2 out]
            n527 = property on="X offset mm" class="DigNum (strict)"() -> ("Value"=w1015:dbl)  [unwired: 2 in, 2 out]
            n528 = property on="Z offset mm" class="DigNum (strict)"() -> ("Value"=w1006:dbl)  [unwired: 2 in, 2 out]
            n529 = Subtract(x=w1032, y=w1024) -> (x-y=w1031:dbl)
            n530 = Subtract(x=w1023, y=w1015) -> (x-y=w1022:dbl)
            n531 = Subtract(x=w1014, y=w1006) -> (x-y=w1013:dbl)
            n532 = property on="Y steps/rev" class="DigNum (strict)"() -> ("Value"=w1026:u32)  [unwired: 2 in, 2 out]
            n533 = property on="X steps/rev" class="DigNum (strict)"() -> ("Value"=w1017:u32)  [unwired: 2 in, 2 out]
            n534 = property on="Z steps/rev" class="DigNum (strict)"() -> ("Value"=w1008:u32)  [unwired: 2 in, 2 out]
            n535 = property on="Y mm/rev" class="DigNum (strict)"() -> ("Value"=w1025:dbl)  [unwired: 2 in, 2 out]
            n536 = property on="X mm/rev" class="DigNum (strict)"() -> ("Value"=w1016:dbl)  [unwired: 2 in, 2 out]
            n537 = property on="Z mm/rev" class="DigNum (strict)"() -> ("Value"=w1007:dbl)  [unwired: 2 in, 2 out]
            n538 = Divide(x=w1031, y=w1025) -> (x/y=w1030:dbl)
            n539 = Divide(x=w1022, y=w1016) -> (x/y=w1021:dbl)
            n540 = Divide(x=w1013, y=w1007) -> (x/y=w1012:dbl)
            n541 = To Double Precision Float(number=w1026) -> (double precision float=w1029:dbl)
            n542 = To Double Precision Float(number=w1017) -> (double precision float=w1020:dbl)
            n543 = To Double Precision Float(number=w1008) -> (double precision float=w1011:dbl)
            n544 = Multiply(x=w1030, y=w1029) -> (x*y=w1028:dbl)
            n545 = Multiply(x=w1021, y=w1020) -> (x*y=w1019:dbl)
            n546 = Multiply(x=w1012, y=w1011) -> (x*y=w1010:dbl)
            n547 = To Long Integer(number=w1028) -> (32bit integer=w1027:i32)
            n548 = To Long Integer(number=w1019) -> (32bit integer=w1018:i32)
            n549 = To Long Integer(number=w1010) -> (32bit integer=w1009:i32)
            n550 = property on="Reset Y Motor Steps" class="DigNum (strict)"("Val(Sgnl)"=w1027) -> ()  [unwired: 2 in, 2 out]
            n551 = property on="Reset X Motor Steps" class="DigNum (strict)"("Val(Sgnl)"=w1018) -> ()  [unwired: 2 in, 2 out]
            n552 = property on="Reset Z Motor Steps" class="DigNum (strict)"("Val(Sgnl)"=w1009) -> ()  [unwired: 2 in, 2 out]
          }
        }
      }
      event "Y Velocity SP step/sec", "X Velocity SP step/sec", "Z Velocity SP step/sec", "Y Step SP", "X Step SP", "Z Step SP": Value Change {
        n553 = event-data() -> ()  [unwired: 1 in, 5 out]
        n554 = property on="X Velocity SP step/sec" class="DigNum (strict)"() -> ("Value"=w1068:i32)  [unwired: 2 in, 2 out]
        n555 = property on="Y Velocity SP step/sec" class="DigNum (strict)"() -> ("Value"=w1074:i32)  [unwired: 2 in, 2 out]
        n556 = property on="Z Velocity SP step/sec" class="DigNum (strict)"() -> ("Value"=w1062:i32)  [unwired: 2 in, 2 out]
        n557 = property on="X steps/rev" class="DigNum (strict)"() -> ("Value"=w1045:u32)  [unwired: 2 in, 2 out]
        n558 = property on="X steps/rev" class="DigNum (strict)"() -> ("Value"=w1066:u32)  [unwired: 2 in, 2 out]
        n559 = property on="Y steps/rev" class="DigNum (strict)"() -> ("Value"=w1053:u32)  [unwired: 2 in, 2 out]
        n560 = property on="Y steps/rev" class="DigNum (strict)"() -> ("Value"=w1072:u32)  [unwired: 2 in, 2 out]
        n561 = property on="Z steps/rev" class="DigNum (strict)"() -> ("Value"=w1037:u32)  [unwired: 2 in, 2 out]
        n562 = property on="Z steps/rev" class="DigNum (strict)"() -> ("Value"=w1060:u32)  [unwired: 2 in, 2 out]
        n563 = property on="X Step SP" class="DigNum (strict)"() -> ("Value"=w1047:i32)  [unwired: 2 in, 2 out]
        n564 = property on="Y Step SP" class="DigNum (strict)"() -> ("Value"=w1055:i32)  [unwired: 2 in, 2 out]
        n565 = property on="Z Step SP" class="DigNum (strict)"() -> ("Value"=w1039:i32)  [unwired: 2 in, 2 out]
        n566 = To Double Precision Float(number=w1047) -> (double precision float=w1048:dbl)
        n567 = To Double Precision Float(number=w1045) -> (double precision float=w1051:dbl)
        n568 = To Double Precision Float(number=w1068) -> (double precision float=w1069:dbl)
        n569 = To Double Precision Float(number=w1066) -> (double precision float=w1071:dbl)
        n570 = To Double Precision Float(number=w1055) -> (double precision float=w1056:dbl)
        n571 = To Double Precision Float(number=w1053) -> (double precision float=w1059:dbl)
        n572 = To Double Precision Float(number=w1074) -> (double precision float=w1075:dbl)
        n573 = To Double Precision Float(number=w1072) -> (double precision float=w1077:dbl)
        n574 = To Double Precision Float(number=w1039) -> (double precision float=w1040:dbl)
        n575 = To Double Precision Float(number=w1037) -> (double precision float=w1043:dbl)
        n576 = To Double Precision Float(number=w1062) -> (double precision float=w1063:dbl)
        n577 = To Double Precision Float(number=w1060) -> (double precision float=w1065:dbl)
        n578 = property on="X mm/rev" class="DigNum (strict)"() -> ("Value"=w1034:dbl)  [unwired: 2 in, 2 out]
        n579 = property on="Y mm/rev" class="DigNum (strict)"() -> ("Value"=w1033:dbl)  [unwired: 2 in, 2 out]
        n580 = property on="Z mm/rev" class="DigNum (strict)"() -> ("Value"=w1035:dbl)  [unwired: 2 in, 2 out]
        n581 = Divide(x=w1048, y=w1051) -> (x/y=w1050:dbl)
        n582 = Divide(x=w1069, y=w1071) -> (x/y=w1070:dbl)
        n583 = Divide(x=w1056, y=w1059) -> (x/y=w1058:dbl)
        n584 = Divide(x=w1075, y=w1077) -> (x/y=w1076:dbl)
        n585 = Divide(x=w1040, y=w1043) -> (x/y=w1042:dbl)
        n586 = Divide(x=w1063, y=w1065) -> (x/y=w1064:dbl)
        n587 = property on="X offset mm" class="DigNum (strict)"() -> ("Value"=w1044:dbl)  [unwired: 2 in, 2 out]
        n588 = property on="Y offset mm" class="DigNum (strict)"() -> ("Value"=w1052:dbl)  [unwired: 2 in, 2 out]
        n589 = property on="Z offset mm" class="DigNum (strict)"() -> ("Value"=w1036:dbl)  [unwired: 2 in, 2 out]
        n590 = Multiply(x=w1050, y=w1034) -> (x*y=w1049:dbl)
        n591 = Multiply(x=w1070, y=w1034) -> (x*y=w1067:dbl)
        n592 = Multiply(x=w1058, y=w1033) -> (x*y=w1057:dbl)
        n593 = Multiply(x=w1076, y=w1033) -> (x*y=w1073:dbl)
        n594 = Multiply(x=w1042, y=w1035) -> (x*y=w1041:dbl)
        n595 = Multiply(x=w1064, y=w1035) -> (x*y=w1061:dbl)
        n596 = property on="X Velocity MV mm/sec" class="DigNum (strict)"("Val(Sgnl)"=w1067) -> ()  [unwired: 2 in, 2 out]
        n597 = property on="Y Velocity MV mm/sec" class="DigNum (strict)"("Val(Sgnl)"=w1073) -> ()  [unwired: 2 in, 2 out]
        n598 = property on="Z Velocity MV mm/sec" class="DigNum (strict)"("Val(Sgnl)"=w1061) -> ()  [unwired: 2 in, 2 out]
        n599 = Add(x=w1049, y=w1044) -> (x+y=w1046:dbl)
        n600 = Add(x=w1057, y=w1052) -> (x+y=w1054:dbl)
        n601 = Add(x=w1041, y=w1036) -> (x+y=w1038:dbl)
        n602 = property on="X Position MV mm" class="DigNum (strict)"("Val(Sgnl)"=w1046) -> ()  [unwired: 2 in, 2 out]
        n603 = property on="Y Position MV mm" class="DigNum (strict)"("Val(Sgnl)"=w1054) -> ()  [unwired: 2 in, 2 out]
        n604 = property on="Z Position MV mm" class="DigNum (strict)"("Val(Sgnl)"=w1038) -> ()  [unwired: 2 in, 2 out]
      }
      event Application Instance Close? {
        n605 = event-data() -> ()  [unwired: 1 in, 4 out]
        n606 = event-data() -> ()  [unwired: 3 in, 1 out]
      }
      event "Stop": Mouse Down {
        n607 = event-data() -> ()  [unwired: 1 in, 7 out]
        n608 = flat-sequence {
          tunnel: [w1099] -> w1087
          tunnel: [w1098] -> w1086
          tunnel: w1085 -> [w1100]
          tunnel: w1084 -> [w1097]
          frame #0 {
            n609 = call "Applied Send Command.vi"("error in (no error)"=w1097, "Command"=T1."Stop", "VISA resource name"=w1100) -> ("error out"=w1098:errorcluster, "VISA resource name out"=w1099:refnum<visa-resource-name>)  [unwired: 4 in, 1 out]
          }
        }
        n610 = flat-sequence {
          tunnel: w1091 -> [w1103]
          tunnel: w1090 -> [w1102]
          tunnel: [w1104] -> w1089
          tunnel: [w1105] -> w1088
          frame #0 {
            n611 = call "Applied Send Command.vi"("error in (no error)"=w1102, "Command"=T1."Stop", "VISA resource name"=w1103) -> ("error out"=w1105:errorcluster, "VISA resource name out"=w1104:refnum<visa-resource-name>)  [unwired: 4 in, 1 out]
          }
        }
        n612 = flat-sequence {
          tunnel: [w1094] -> w1081
          tunnel: [w1095] -> w1080
          tunnel: w1083 -> [w1092]
          tunnel: w1082 -> [w1093]
          frame #0 {
            n613 = call "Applied Send Command.vi"("error in (no error)"=w1093, "Command"=T1."Stop", "VISA resource name"=w1092) -> ("error out"=w1095:errorcluster, "VISA resource name out"=w1094:refnum<visa-resource-name>)  [unwired: 4 in, 1 out]
          }
        }
      }
      event "Reset": Mouse Down {
        n614 = event-data() -> ()  [unwired: 1 in, 7 out]
        n615 = flat-sequence {
          tunnel: [w1126] -> w1112
          tunnel: w1113 -> [w1128]
          tunnel: [w1127] -> w1111
          tunnel: w1114 -> [w1129]
          frame #0 {
            n616 = property on="Reset X Motor Steps" class="DigNum (strict)"() -> ("Value"=w1132:i32)  [unwired: 2 in, 2 out]
            n617 = Number To Decimal String(number=w1132) -> (decimal integer string=w1130:string)  [unwired: 1 in]
            n618 = call "Applied Send Command.vi"("error in (no error)"=w1128, "Extra"=w1130, "Command"=T1."Set ABS Position", "VISA resource name"=w1129) -> ("error out"=w1127:errorcluster, "VISA resource name out"=w1126:refnum<visa-resource-name>)  [unwired: 3 in, 1 out]
          }
        }
        n619 = flat-sequence {
          tunnel: w1118 -> [w1137]
          tunnel: w1117 -> [w1134]
          tunnel: [w1136] -> w1116
          tunnel: [w1135] -> w1115
          frame #0 {
            n620 = property on="Reset Y Motor Steps" class="DigNum (strict)"() -> ("Value"=w1139:i32)  [unwired: 2 in, 2 out]
            n621 = Number To Decimal String(number=w1139) -> (decimal integer string=w1138:string)  [unwired: 1 in]
            n622 = call "Applied Send Command.vi"("error in (no error)"=w1134, "Extra"=w1138, "Command"=T1."Set ABS Position", "VISA resource name"=w1137) -> ("error out"=w1135:errorcluster, "VISA resource name out"=w1136:refnum<visa-resource-name>)  [unwired: 3 in, 1 out]
          }
        }
        n623 = flat-sequence {
          tunnel: [w1124] -> w1108
          tunnel: [w1123] -> w1107
          tunnel: w1110 -> [w1121]
          tunnel: w1109 -> [w1122]
          frame #0 {
            n624 = property on="Reset Z Motor Steps" class="DigNum (strict)"() -> ("Value"=w1125:i32)  [unwired: 2 in, 2 out]
            n625 = Number To Decimal String(number=w1125) -> (decimal integer string=w1119:string)  [unwired: 1 in]
            n626 = call "Applied Send Command.vi"("error in (no error)"=w1122, "Extra"=w1119, "Command"=T1."Set ABS Position", "VISA resource name"=w1121) -> ("error out"=w1123:errorcluster, "VISA resource name out"=w1124:refnum<visa-resource-name>)  [unwired: 3 in, 1 out]
          }
        }
      }
    }
    n627 = case shown="False" "Reset Jog counts" {
      frame False {
      }
      frame True {
        w297 = 0
        n628 = local write "FY Jog counts"(w297) -> ()
        n629 = local write "FZ Jog counts"(w297) -> ()
        n630 = local write "FX Jog counts"(w297) -> ()
      }
    }
    n631 = flat-sequence {
      frame #0 {
        w767 = 10 ("number of samples")
        n632 = Build Array("Dev 5 Voltage SW") -> (w766:bool[])
        n633 = Boolean To (0,1)(Boolean="Dev 5 Voltage SW") -> (0, 1=w764:i16)
        n634 = call "DAQ AI0"("number of samples"=w767) -> ("data"=w772:dynamicdata)  [unwired: 16 in, 2 out]
        n635 = Multiply(x=w764, y=i16 5) -> (x*y=w762:i16)
        n636 = call "DAQ P1.7"("data"=w766) -> ()  [unwired: 17 in, 2 out]
        n637 = call "Convert from Dynamic Data2"("Dynamic Data Type"=w772) -> ("Array"=w773:dbl[])  [unwired: 3 in]
        n638 = Add Array Elements(numeric array=w773) -> (sum=w771:dbl)
        n639 = Divide(x=w771, y=w767) -> (x/y=w770:dbl)
        n640 = Multiply(x=w762, y=0.8) -> (x*y=w768:dbl)
        n641 = Absolute Value(x=w770) -> (abs(x)=w761:dbl)
        "Dev5 Voltage PV" <- w761
        n642 = Greater?(x=w761, y=w768) -> (0:w774:bool)
        n643 = call-poly <userlib>:"CaLabPut.vi"("Value"=w761, "PV Name"="SSE:Tsample") -> ()  [unwired: 6 in, 4 out]
        n644 = case shown="True" "Crash Override" {
          tunnel: [w777 TRUE] -> w775
          tunnel: w774 -> [w777 _]
          frame False {
          }
          frame True {
          }
        }
        "Isolated from GND?" <- w775
      }
    }
  }
  n645 = flat-sequence {
    tunnel: w37 -> [w1141]
    tunnel: w36 -> [w1140]
    tunnel: [w1152] -> w21
    frame #0 {
      # "GET CURRENT POSITION"
      n646 = call "Applied Send Command.vi"("error in (no error)"=w1140, "Extra"="", "Command"=T1."Immediate Position?", "VISA resource name"=w1141) -> ("error out"=w1142:errorcluster, "read buffer"=w1147:string, "VISA resource name out"=w1143:refnum<visa-resource-name>)  [unwired: 3 in]
      n647 = call "Applied Send Command.vi"("error in (no error)"=w1142, "Command"=T1."Stop & Kill Buffer", "VISA resource name"=w1143) -> ("error out"=w1149:errorcluster, "VISA resource name out"=w1150:refnum<visa-resource-name>)  [unwired: 4 in, 1 out]
      n648 = Hexadecimal String To Number(string=w1147, offset=3) -> (number=w1144:u32)  [unwired: 1 in, 1 out]
      n649 = VISA Close(VISA resource name=w1150, error in (no error)=w1149) -> ()  [unwired: 1 out]
      n650 = To Long Integer(number=w1144) -> (32bit integer=w1152:i32)
    }
  }
  n651 = flat-sequence {
    tunnel: w23 -> [w1155]
    tunnel: w22 -> [w1154]
    tunnel: [w1153] -> w20
    frame #0 {
      # "GET CURRENT POSITION"
      n652 = call "Applied Send Command.vi"("error in (no error)"=w1154, "Extra"="", "Command"=T1."Immediate Position?", "VISA resource name"=w1155) -> ("error out"=w1156:errorcluster, "read buffer"=w1161:string, "VISA resource name out"=w1157:refnum<visa-resource-name>)  [unwired: 3 in]
      n653 = call "Applied Send Command.vi"("error in (no error)"=w1156, "Command"=T1."Stop & Kill Buffer", "VISA resource name"=w1157) -> ("error out"=w1163:errorcluster, "VISA resource name out"=w1164:refnum<visa-resource-name>)  [unwired: 4 in, 1 out]
      n654 = Hexadecimal String To Number(string=w1161, offset=3) -> (number=w1158:u32)  [unwired: 1 in, 1 out]
      n655 = VISA Close(VISA resource name=w1164, error in (no error)=w1163) -> ()  [unwired: 1 out]
      n656 = To Long Integer(number=w1158) -> (32bit integer=w1153:i32)
    }
  }
  n657 = flat-sequence {
    tunnel: w25 -> [w1167]
    tunnel: w24 -> [w1166]
    tunnel: [w1168] -> w19
    frame #0 {
      # "GET CURRENT POSITION"
      n658 = call "Applied Send Command.vi"("error in (no error)"=w1166, "Extra"="", "Command"=T1."Immediate Position?", "VISA resource name"=w1167) -> ("error out"=w1169:errorcluster, "read buffer"=w1174:string, "VISA resource name out"=w1170:refnum<visa-resource-name>)  [unwired: 3 in]
      n659 = call "Applied Send Command.vi"("error in (no error)"=w1169, "Command"=T1."Stop & Kill Buffer", "VISA resource name"=w1170) -> ("error out"=w1176:errorcluster, "VISA resource name out"=w1177:refnum<visa-resource-name>)  [unwired: 4 in, 1 out]
      n660 = Hexadecimal String To Number(string=w1174, offset=3) -> (number=w1171:u32)  [unwired: 1 in, 1 out]
      n661 = VISA Close(VISA resource name=w1177, error in (no error)=w1176) -> ()  [unwired: 1 out]
      n662 = To Long Integer(number=w1171) -> (32bit integer=w1168:i32)
    }
  }
  n663 = flat-sequence {
    tunnel: w21 -> [w1183]
    tunnel: w20 -> [w1182]
    tunnel: w19 -> [w1181]
    frame #0 {
      n664 = Build Array(w1183, w1182, w1181) -> (w1179:i32[])
      n665 = call-poly <vilib>:"Write To Spreadsheet File.vi"("1D data"=w1179, "file path (dialog if empty)"=path "S:/SSE/SCL2/POS.TXT") -> ()  [unwired: 6 in, 1 out]
    }
    frame #1 {
    }
  }
